vi "MainPr(Calculation)-37.vi"() -> ()   [LabVIEW 2013]
doc: "Main Program for Tracking\nThis VI Represents Front Panel and Control Buttons for Perform Tracking\nPlease, optimize the front panel for your own monitor resolution and needs"
uses:
  <vilib>/Utility/file.llb/Write To Spreadsheet File (DBL).vi
  <vilib>/vision/NI_Vision_Development_Module.lvlib
panel:
  out "error out":errorcluster
  in  "STOP Program":bool
  in  "Front Panel":T1(tab)
  in  "CurFrame":u32 max=9
  in  "Parameter 2":sgl format="%.2f"
  in  "Operator 2":T2(ring)
  out "2nd Movie (now disabled)":T3(plugin-control)
  out "1st Movie":T3(plugin-control)
  in  "Parameter":sgl format="%.2f"
  in  "Operator":T2(ring)
  in  "Index for thresholding 2":u8
  in  "Parameter 3":sgl format="%.2f"
  in  "Operator 3":T2(ring)
  in  "1/2 Channels":bool
  in  "Sigma #2":dbl min=0.1
  in  "Sigma":dbl min=0.1
  in  "Frame2":u32 max=499
  in  "Gray or Binarized?":bool
  out "2nd Movie Processed (now disabled)":T3(plugin-control)
  out "1st Movie Processed":T3(plugin-control)
  in  "Index for thresholding":u8 max=202
  in  "Keep Nega-\ntive Values?":bool
  out "Histogram of LoG \nprocessed image":T4(graph)
  out "Progress":u8(slide) scale=0.0..100.0
  in  "# Frame3":u32 max=499
  in  "Save pics (ex)":bool
  in  "Find ALL objects":bool
  out "Results on 1st Movie":T3(plugin-control)
  out "1st Filtering":T3(plugin-control)
  in  "Try my filters!":bool
  in  "# Erosion":i32=2
  in  "Connectivity":bool=TRUE
  in  "Min  Diam":dbl
  in  "Max  Diam":dbl min=12.0
  in  "Filter Tracks":bool
  out "Tracking progress":u8(slide) scale=0.0..100.0
  in  "Save data":bool
  in  "Save pictures":bool
  in  "Save movies":bool
  in  "Frame":u32 max=499
  in  "Delete Tracs":bool
  out "1st Filtered":T3(plugin-control)
  in  "dR max":dbl min=1.0
  out "1st Filtering (NN)":T3(plugin-control)
  in  "dR min":dbl min=0.0 max=10.0
  out "Raw #":i32
  out "Saved #":i32
  in  "Tracking Procedure":bool
  in  "Min TRK L":i32 min=2 max=498 step=1
  in  "Closing gaps":i32 min=1 max=498 step=1
  in  "% linearity":i32 min=1 max=100 step=1
  in  "Max angle":dbl min=0.0 max=89.0 step=1.0
  in  "Save problem trks":bool
  in  "Save pictures 2":bool
  in  "Delete Tracs 3":bool
  in  "Testing Frame":u32 min=68 max=76
  out "After":T3(plugin-control)
  out "Before":T3(plugin-control)
  in  "Tracks group":i32 min=0 max=515
  in  "Show Distributions":bool
  out "All Path Vel":T5(graph)
  out "All Instant Vel":T5(graph)
  out "mean Instant Vel":dbl format="%#_2g"
  out "StD Instant":dbl format="%#_2g"
  out "mean Path Vel":dbl format="%.2f"
  out "StD Path":dbl format="%.2f"
  in  "Bins":i32=10
  # "Two channels"
  # "*Two channels proce\nssing coming SOON"
  # "One channel"
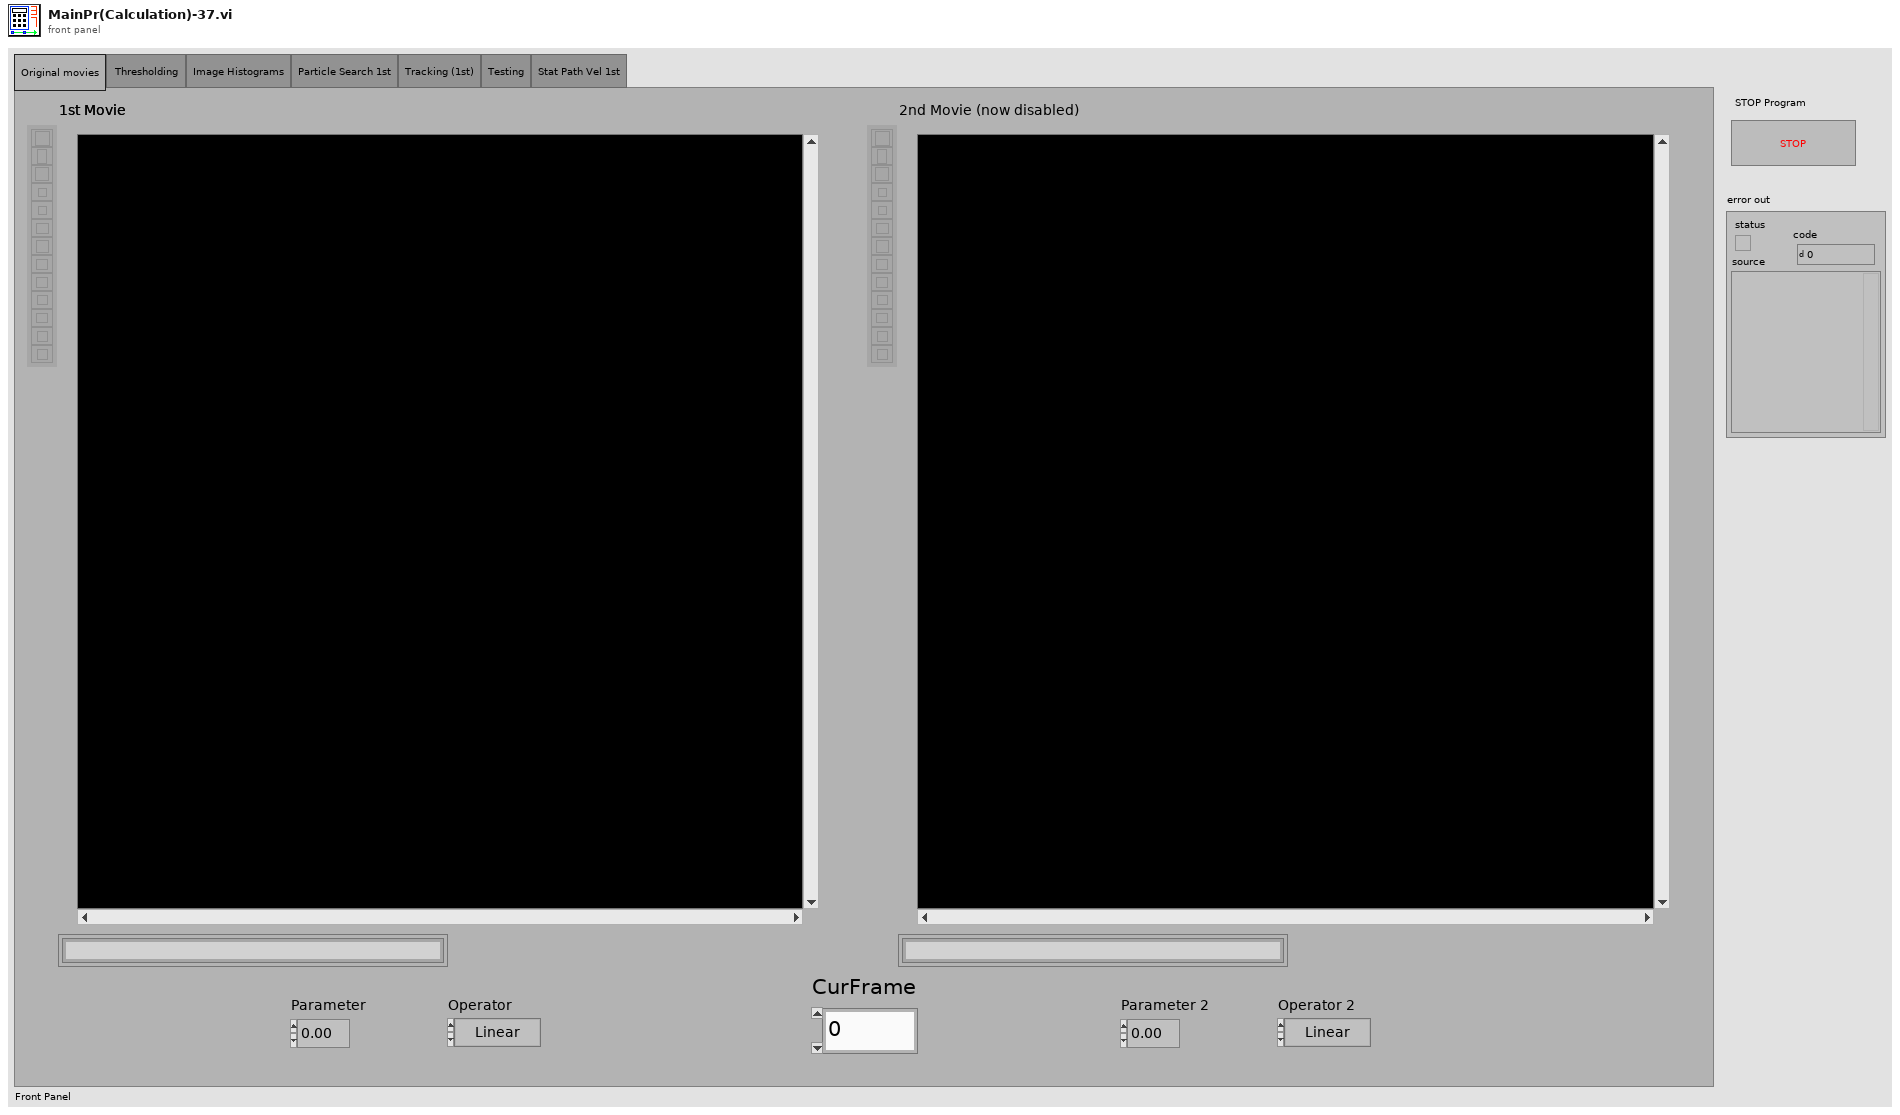
[diagram p1: front panel]
types:
  T1 = enum32{"Original movies", "Thresholding ", "Image Histograms", "Particle Search 1st", "Tracking (1st)", "Testing", "Stat Path Vel 1st"}
  T2 = enum32{"Linear", "Log", "Exp", "Square", "Square root", "Power X", "Power 1/X"}
  T3 = typedef "IMAQ Image.ctl" = refnum<image>
  T4 = cluster{"Starting Value":sgl, "Incremental Value":sgl, "Histogram":u32[]}
  T5 = cluster{"X Values":dbl[], "Histogram: h(x)":i32[]}
  T6 = enum8{"Enabled", "Disabled", "Disabled and Grayed Out"}
  T7 = cluster{"dR min ":dbl, "dR max ":dbl, "Closing gaps":i32, "Min TRK L":i32, "% linearity":i32, "Max angle":dbl, "Tracking progress":refnum<vi>}
  T8 = typedef "Image Type" = u32
  T9 = typedef "IMAQ AVI2 Refnum.ctl" = refnum<k20>
  T10 = cluster{"Intensity #1":sgl, "Operator #1":enum32{"Linear", "Log", "Exp", "Square", "Square root", "Power X", "Power 1/X"}, "Intensity #2":sgl, "Operator #2":enum32{"Linear", "Log", "Exp", "Square", "Square root", "Power X", "Power 1/X"}, "Sigma #1":dbl, "Sigma #2":dbl, "Index for \nthresholding":u8, "Index for \nthresholding 2":u8}
  T11 = typedef "Particle Parameters" = i32
  T12 = cluster{"X,Y":dbl[][], "Areas particles":dbl[][], "Particle Fil Setups":cluster{"Erosion":i32, "Connectivity ":bool, "Type of particle filter":cluster{"Measurement Parameter":T11, "Min  Diam":dbl, "Max  Diam":dbl, "Range":bool, "Range":bool}[]}, "Tracks, Coordinates":cluster{"(X,Y) Unmoved":dbl[][], "(X,Y,dX,dY) Dur 1 Frame":dbl[][], "(X,Y,dX,dY) W/t Problems":dbl[][], "(X,Y,dX,dY) NN filtered":dbl[][], "(X,Y,dX,dY) TH filtered":dbl[][], "Tracks":cluster{"Tracks":dbl[], "Start Pos":i32}[], "Tracks w/t Problems":cluster{"Tracks":dbl[], "Start Pos":i32}[]}}
  T13 = cluster{"Instant Vel 1st":dbl[], "Path Vel 1st ":dbl[], "Instant Vel 2nd  ":dbl[], "Path Vel 2nd":dbl[], "Time Measurments (Moving)":i32[], "Time Measurments (Unmoving) ":i16[]}
  T14 = cluster{"Before Grouped Tracks":cluster{"Tracks":dbl[][], "Start Pos":i32[], "Dot Statuses":i16[][]}[], "After Grouped Tracks":cluster{"Tracks":dbl[][], "Start Pos":i32[], "Dot Statuses":i16[][]}[], "Current\nGroup":i32}
  T15 = cluster{"Erosion":i32, "Connectivity ":bool, "Type of particle filter":cluster{"Measurement Parameter":T11, "Min  Diam":dbl, "Max  Diam":dbl, "Range":bool, "Range":bool}[]}
  T16 = cluster{"(X,Y) Unmoved":dbl[][], "(X,Y,dX,dY) Dur 1 Frame":dbl[][], "(X,Y,dX,dY) W/t Problems":dbl[][], "(X,Y,dX,dY) NN filtered":dbl[][], "(X,Y,dX,dY) TH filtered":dbl[][], "Tracks":cluster{"Tracks":dbl[], "Start Pos":i32}[], "Tracks w/t Problems":cluster{"Tracks":dbl[], "Start Pos":i32}[]}
  T17 = cluster{"Measurement Parameter":T11, "Min  Diam":dbl, "Max  Diam":dbl, "Range":bool, "Range":bool}[]
  T18 = cluster{"Points (X,Y)":dbl[], "Areas of points (X,Y)":dbl[]}[]
  T19 = cluster{"Points (X,Y)":dbl[], "Areas of points (X,Y)":dbl[]}
  T20 = cluster{"Area":dbl, "Number of Holes":dbl, "Bounding Rect":cluster{"Left":dbl, "Top":dbl, "Right":dbl, "Bottom":dbl}, "Center of Mass":cluster{"X":dbl, "Y":dbl}, "Orientation":dbl, "Dimensions":cluster{"Width":dbl, "Height":dbl}}[]
  T21 = cluster{"Tracks W/T Problems":dbl[], "Start Pos":i32}[]
  T22 = cluster{"Tracks":dbl[][], "Start Pos":i32[], "Dot Statuses":i16[][]}[]
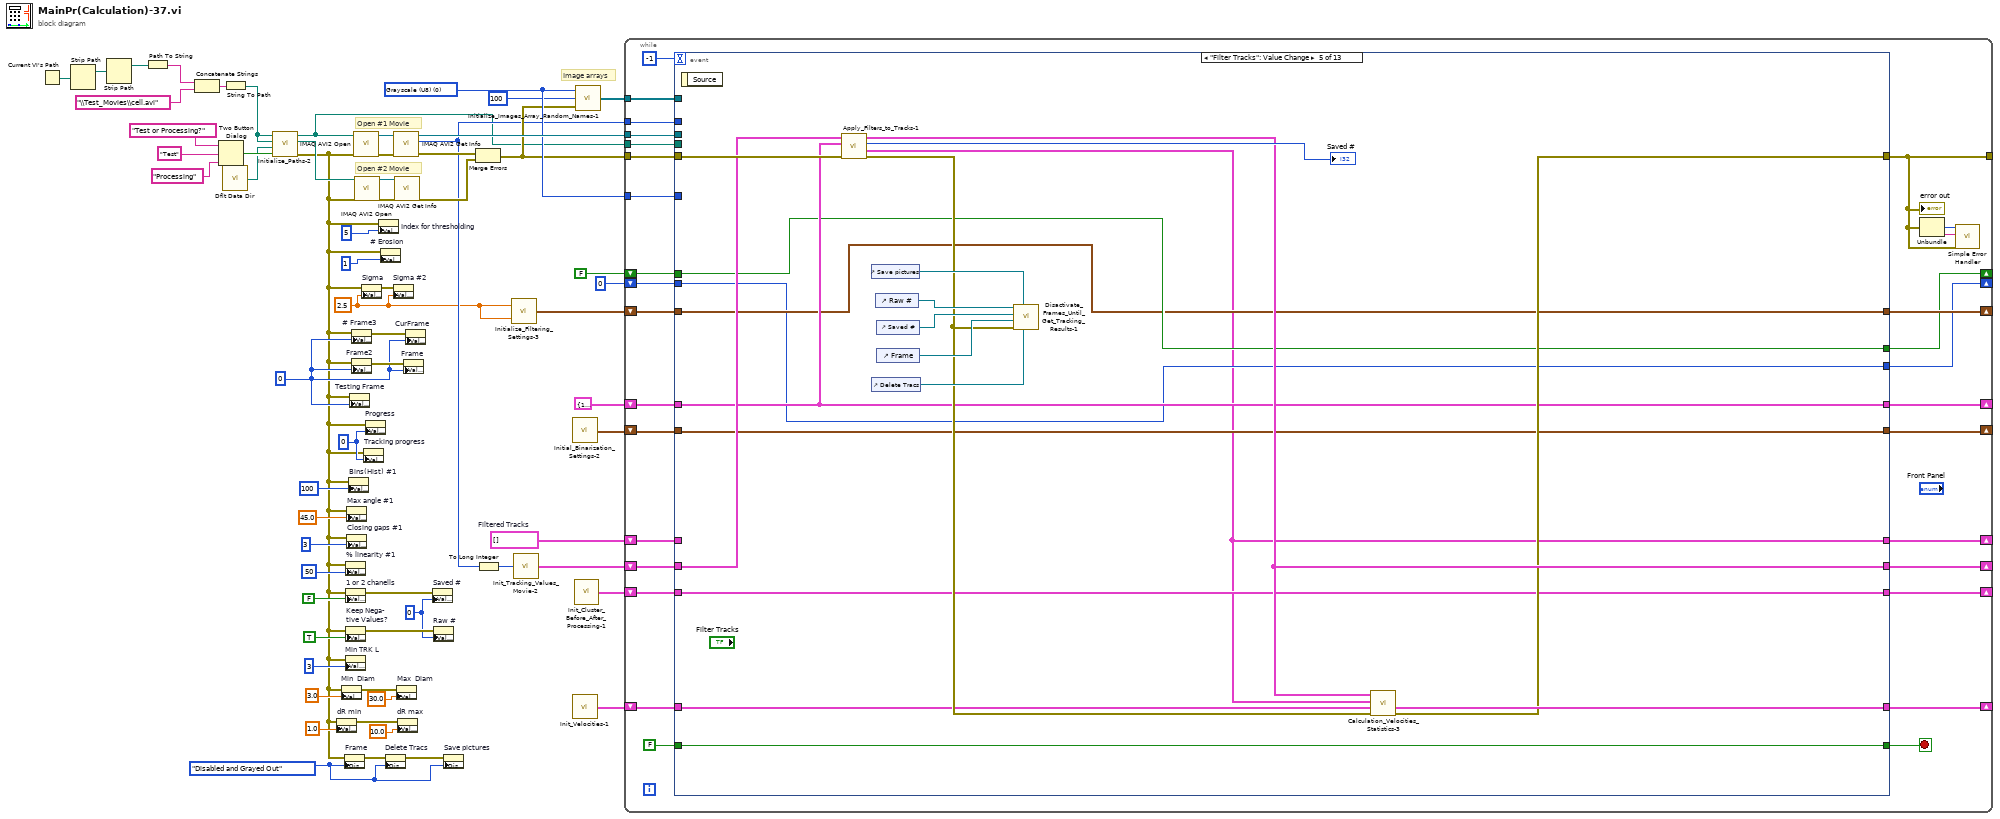
[diagram p0: block diagram]
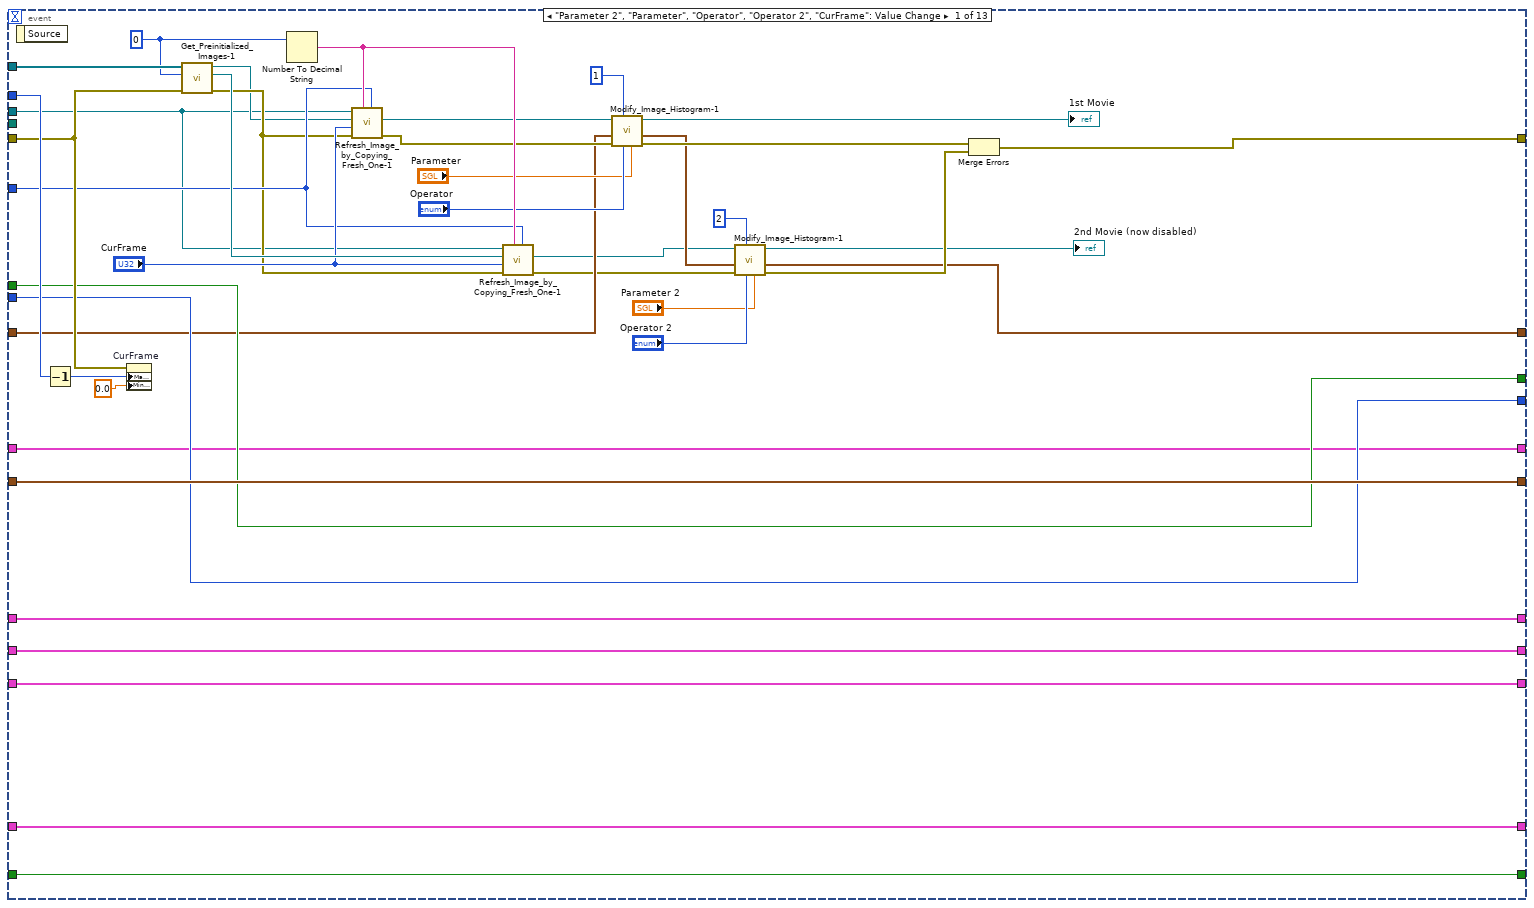
[diagram p2: hidden frame]
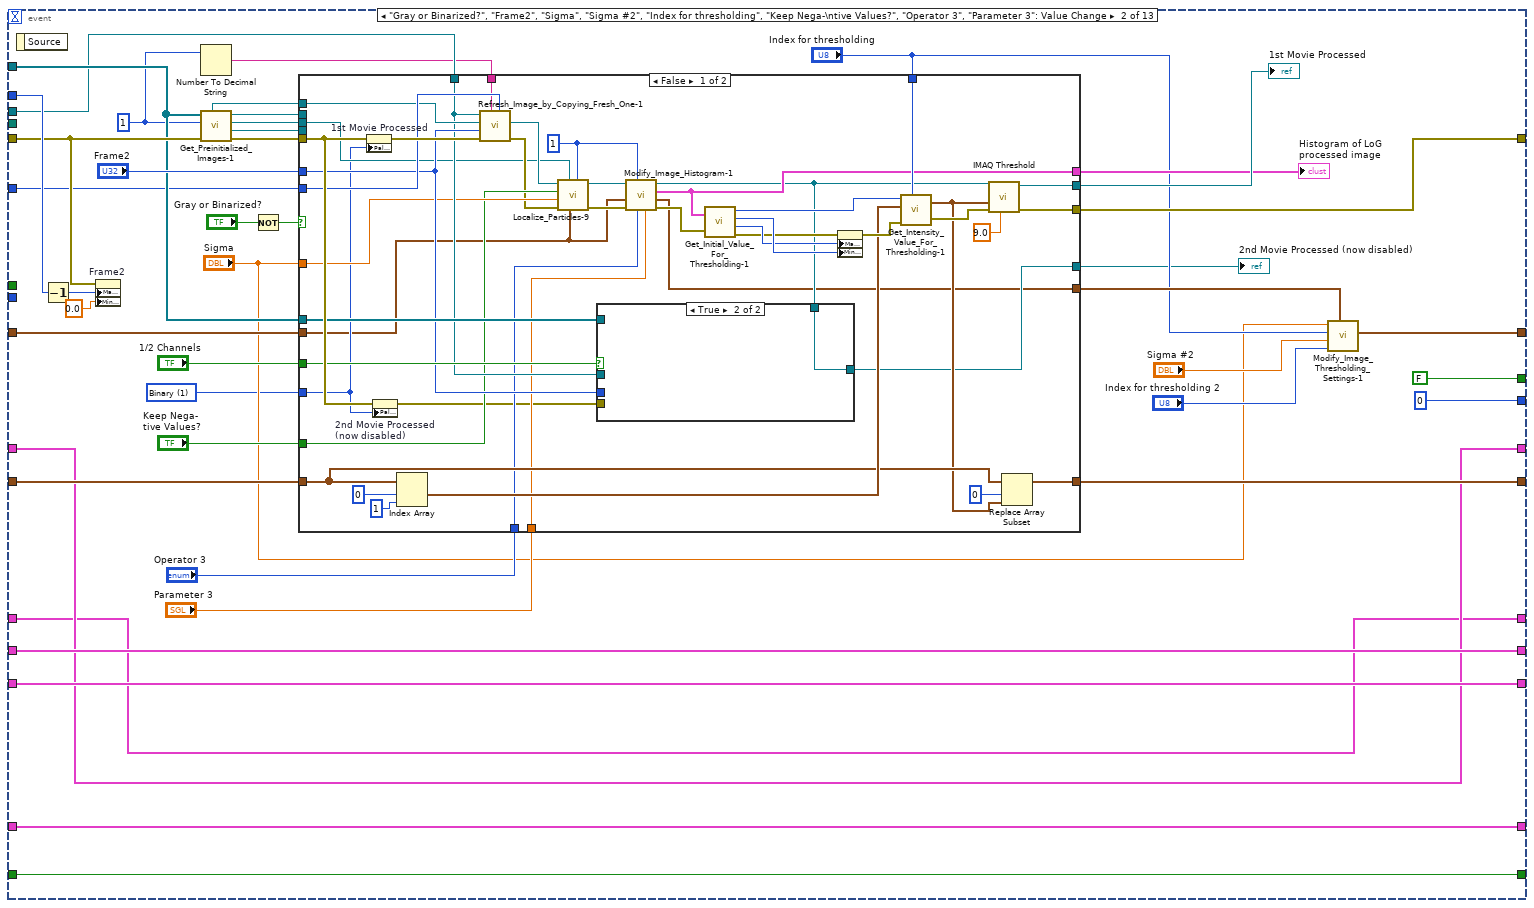
[diagram p3: hidden frame]
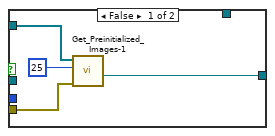
[diagram p4: hidden frame]
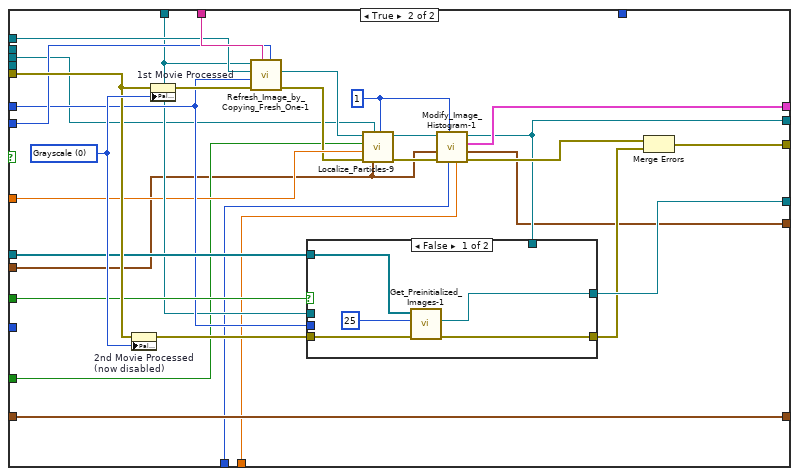
[diagram p5: hidden frame]
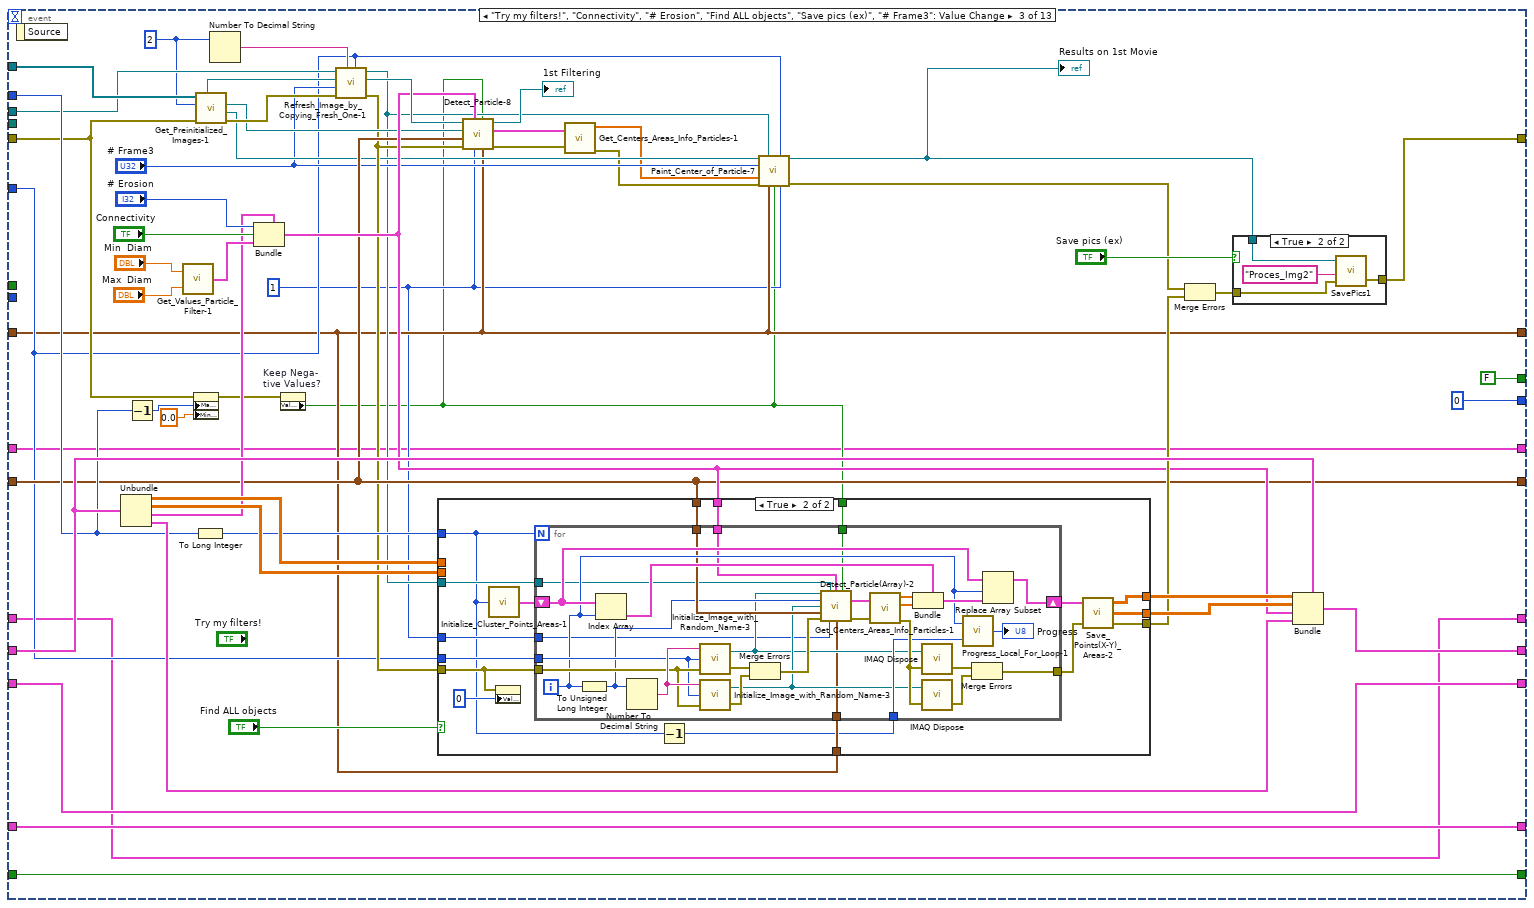
[diagram p7: hidden frame]
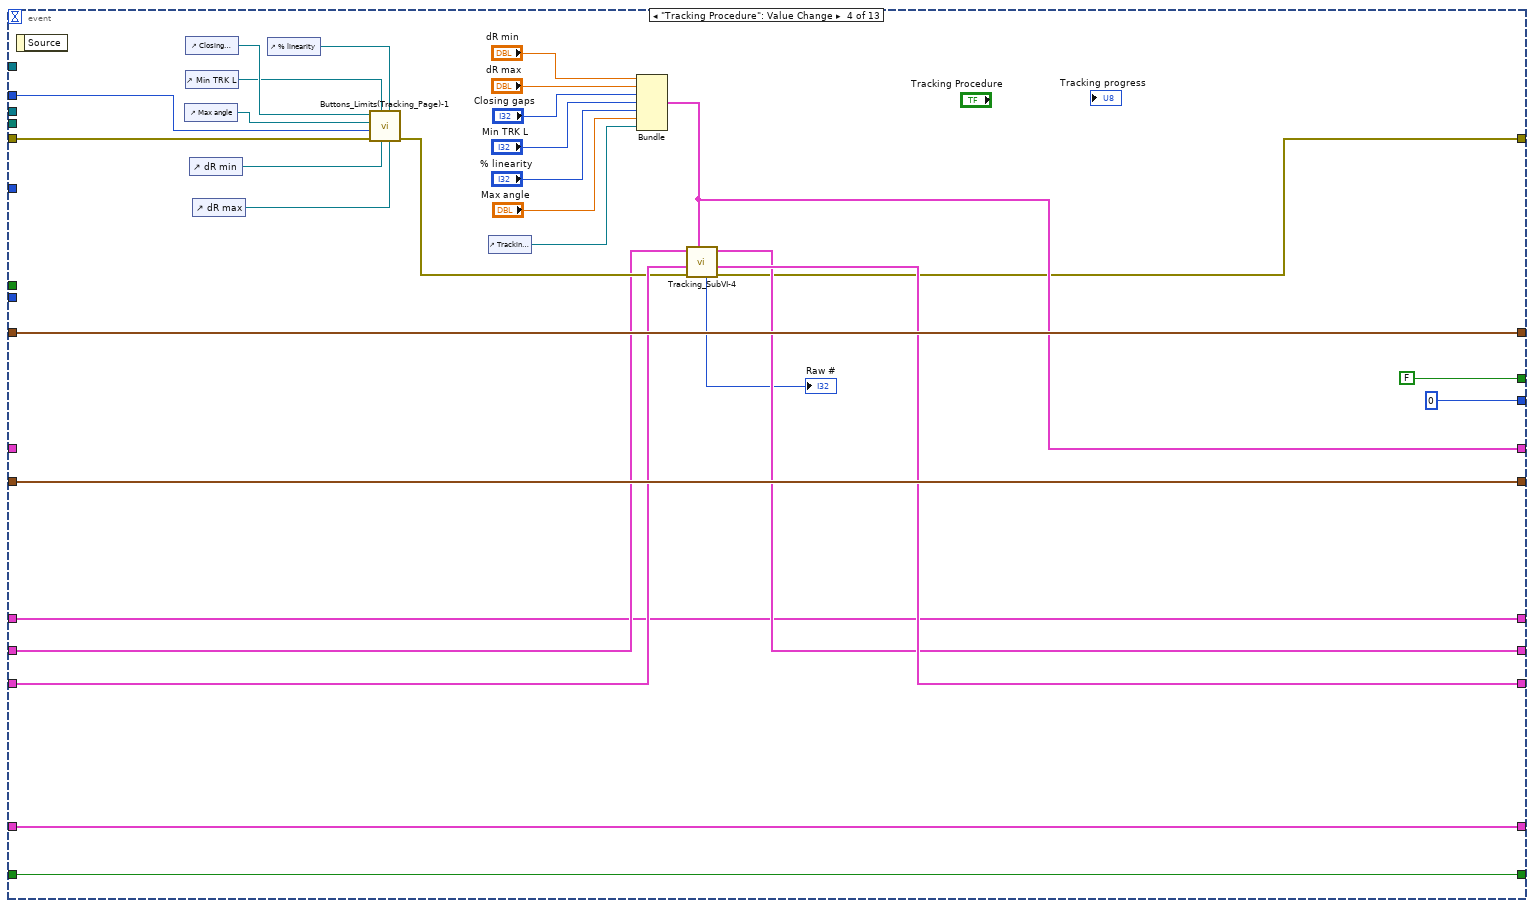
[diagram p10: hidden frame]
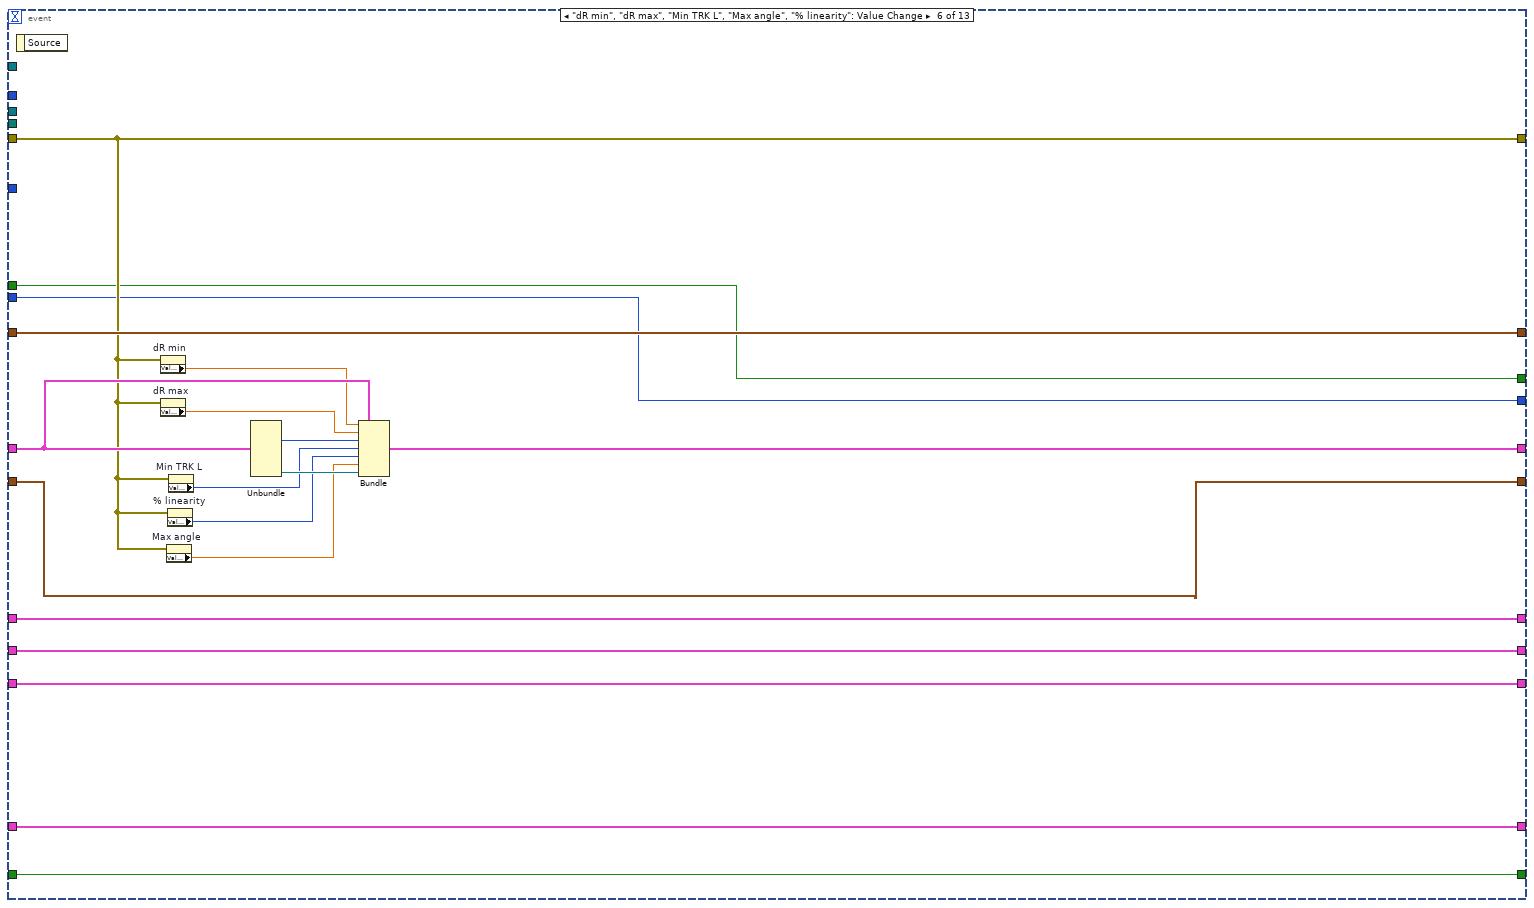
[diagram p11: hidden frame]
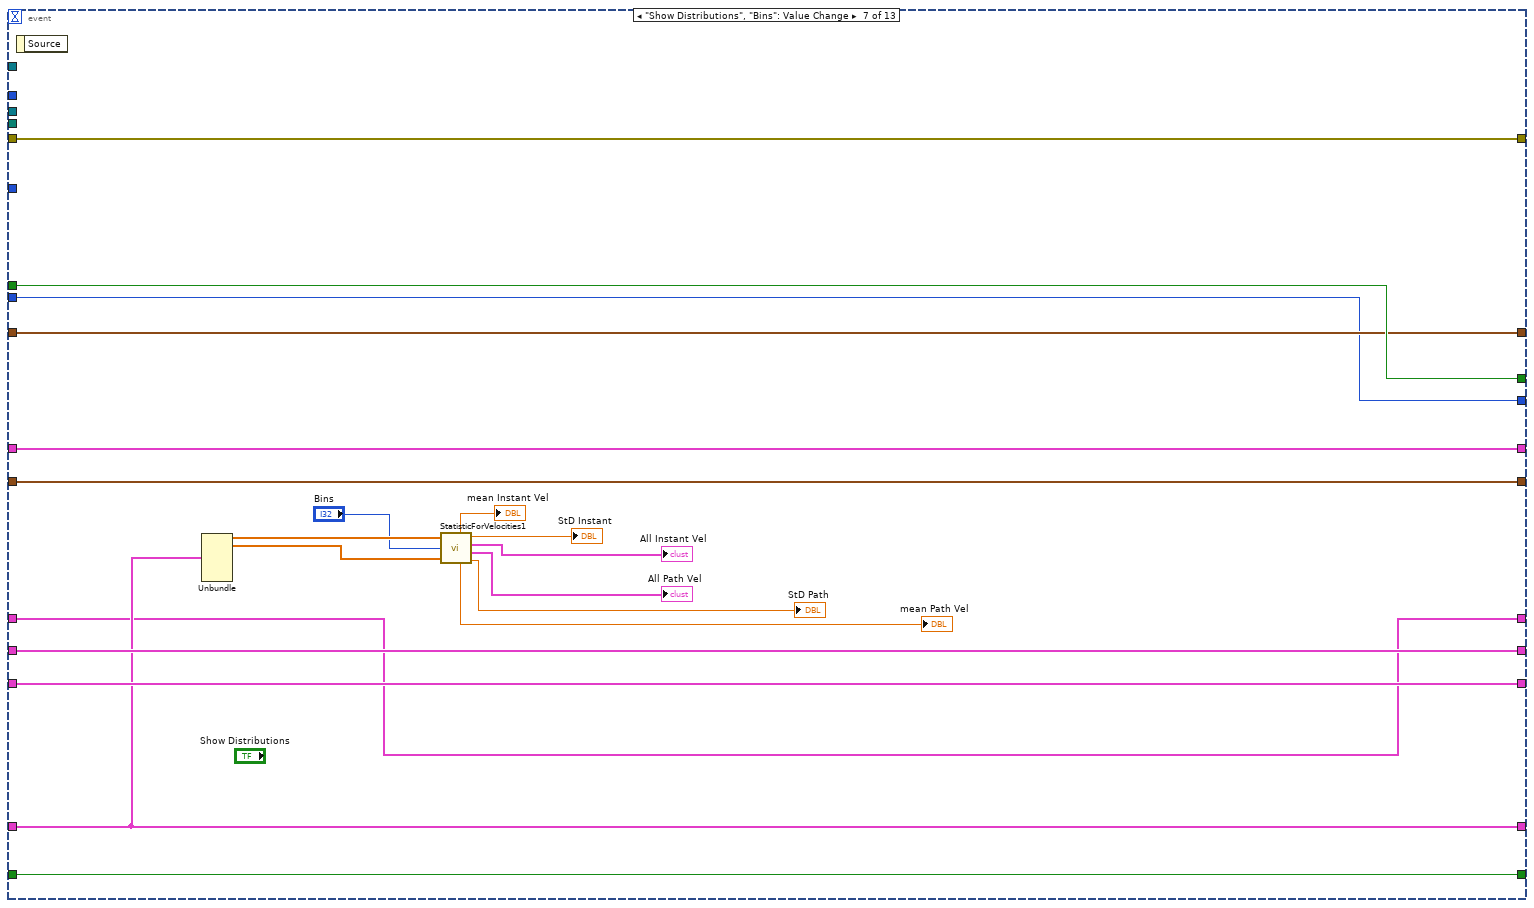
[diagram p12: hidden frame]
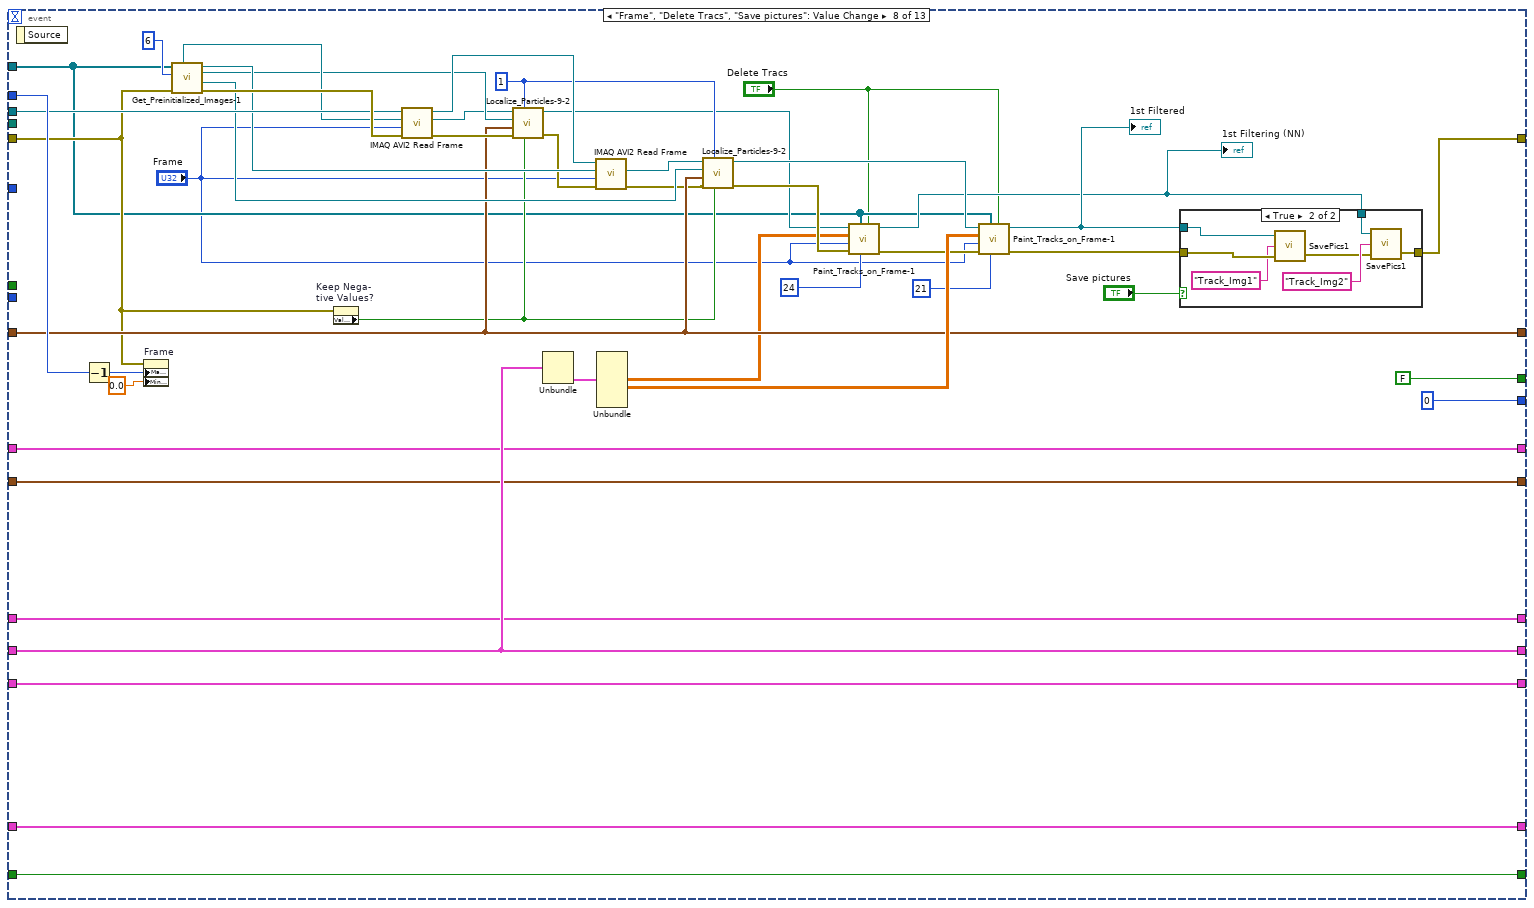
[diagram p13: hidden frame]
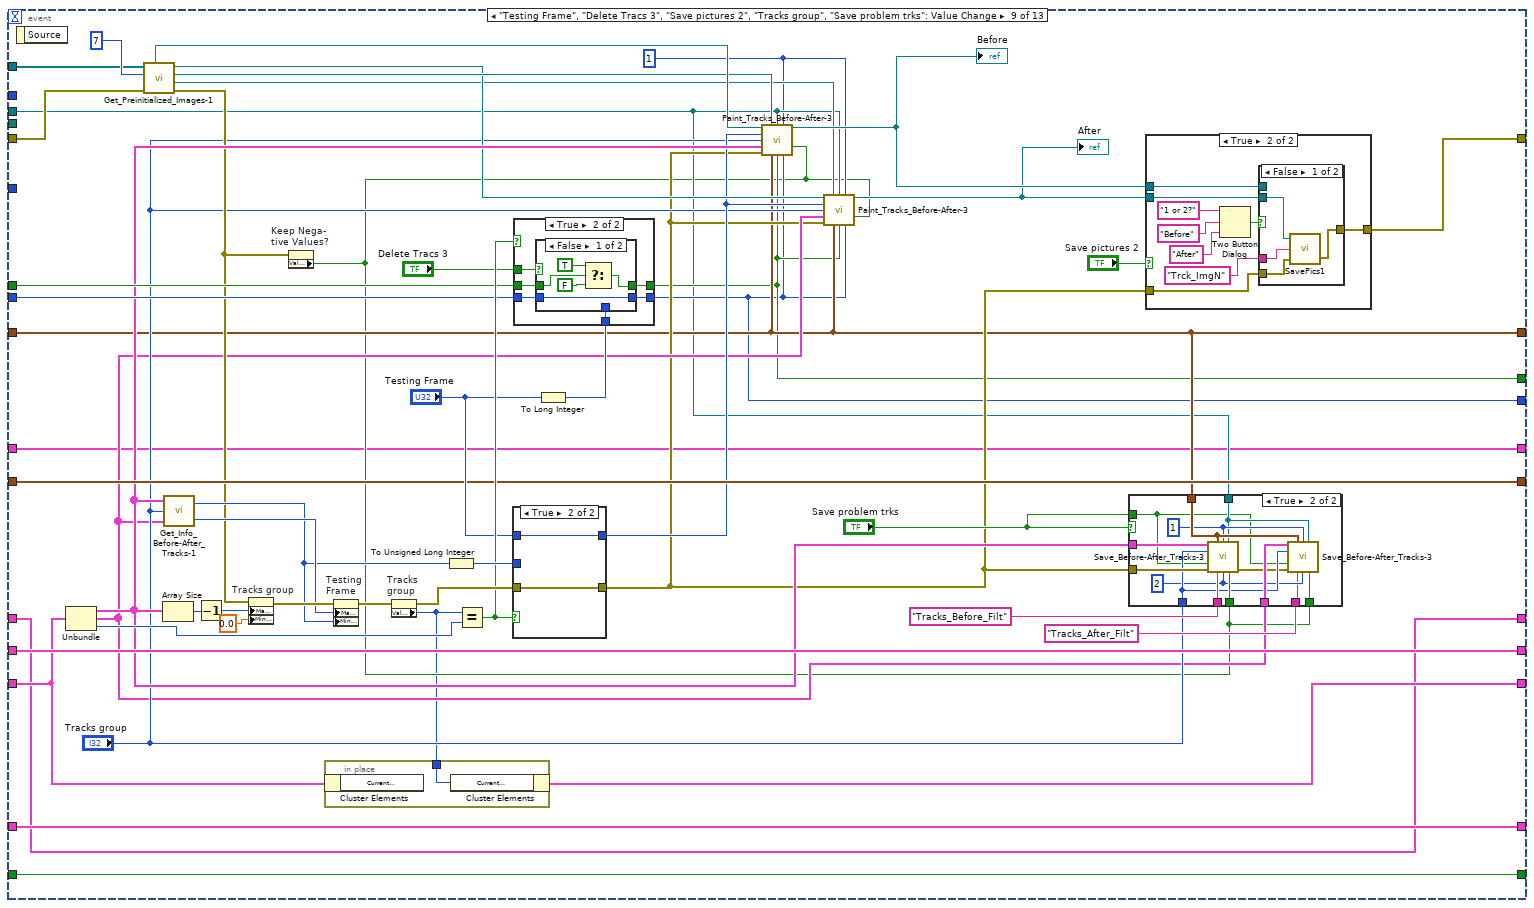
[diagram p15: hidden frame]
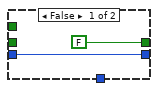
[diagram p16: hidden frame]
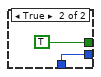
[diagram p17: hidden frame]
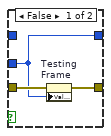
[diagram p19: hidden frame]
diagram:
  w1 = 0 ("Saved #")
  w4 = cluster{"Tracks":dbl[], "Start Pos":i32}[] []  # Filtered Tracks
  w5 = T6."Disabled and Grayed Out" ("Disabled")
  w14 = u32 0 ("Testing Frame")
  w27 = u8 0 ("Progress")
  w26 = 2.5 ("Sigma")
  w38 = T8 0 items=["Grayscale (U8)", "Grayscale (I16)", "Grayscale (SGL)", "Complex (CSG)", "RGB (U32)", "HSL (U32)", "RGB (U64)", "Grayscale (U16)"] ("Image Type")
  # "Image arrays"
  # "Open #2 Movie"
  # "Open #1 Movie"
  n1 = Current VI's Path() -> (path=w18:path)
  n2 = Strip Path(path=w18) -> (stripped path=w13:path)  [unwired: 1 out]
  n3 = Strip Path(path=w13) -> (stripped path=w12:path)  [unwired: 1 out]
  n4 = Path To String(path=w12) -> (string=w23:string)
  n5 = Concatenate Strings(w23, "\\Test_Movies\\cell.avi" ("string")) -> (w20:string)
  n6 = Two Button Dialog(message="Test or Processing?", 1:"Processing" ("F button name (\"Cancel\")"), 2:"Test" ("T button name (\"OK\")")) -> (T button?=w33:bool)
  n7 = call <vilib>:"Dflt Data Dir.vi"() -> ("App:Default Data Directory"=w21:path)
  n8 = String To Path(string=w20) -> (path=w19:path)
  n9 = call "Initialize_Paths-2.vi"("Test or Processing?"=w33, "start path"=w21, "AVI File Path #2"=w19, "AVI File Path #1"=w19) -> ("ERROR OUT"=w10:errorcluster, "AVI File Path #2 OUT"=w32:path, "AVI File Path #1 OUT"=w17:path)  [unwired: 1 out]
  n10 = property on="dR min" class="DigNum (strict)"(error in=w10, "Value"=1.0 ("dR min")) -> (error out=w42:errorcluster)  [unwired: 1 in, 1 out]
  n11 = property on="Min  Diam" class="DigNum (strict)"(error in=w10, "Value"=3.0 ("Min  Diam")) -> (error out=w45:errorcluster)  [unwired: 1 in, 1 out]
  n12 = property on="Frame" class="DigNum (strict)"(error in=w10, "DisabledEnum"=w5) -> (error out=w7:errorcluster)  [unwired: 1 in, 1 out]
  n13 = property on="Min TRK L" class="DigNum (strict)"(error in=w10, "Value"=3 ("Min TRK L")) -> ()  [unwired: 1 in, 2 out]
  n14 = property on="% linearity #1" class="DigNum (strict)"(error in=w10, "Value"=50 ("% linearity")) -> ()  [unwired: 1 in, 2 out]
  n15 = property on="1 or 2 chanells" class="Bool (strict)"(error in=w10, "Value"=FALSE) -> (error out=w3:errorcluster)  [unwired: 1 in, 1 out]
  n16 = property on="Keep Nega-\ntive Values?" class="Bool (strict)"(error in=w10, "Value"=TRUE ("Keep Nega-\ntive Values?")) -> (error out=w2:errorcluster)  [unwired: 1 in, 1 out]
  n17 = property on="Max angle #1" class="DigNum (strict)"(error in=w10, "Value"=45.0 ("Max angle")) -> ()  [unwired: 1 in, 2 out]
  n18 = property on="Closing gaps #1" class="DigNum (strict)"(error in=w10, "Value"=3 ("Closing gaps")) -> ()  [unwired: 1 in, 2 out]
  n19 = property on="Bins(Hist) #1" class="DigNum (strict)"(error in=w10, "Value"=100 ("Intervals")) -> ()  [unwired: 1 in, 2 out]
  n20 = property on="Testing Frame" class="DigNum (strict)"(error in=w10, "Value"=w14) -> ()  [unwired: 1 in, 2 out]
  n21 = property on="# Frame3" class="DigNum (strict)"(error in=w10, "Value"=w14) -> (error out=w16:errorcluster)  [unwired: 1 in, 1 out]
  n22 = property on="Frame2" class="DigNum (strict)"(error in=w10, "Value"=w14) -> (error out=w15:errorcluster)  [unwired: 1 in, 1 out]
  n23 = call "IMAQ AVI2 Open"("error in (no error)"=w10, "AVI File Path"=w17) -> ("error out"=w63:errorcluster, "AVI Refnum"=w64:T9)  [unwired: 8 in]
  n24 = call "IMAQ AVI2 Open"("error in (no error)"=w10, "AVI File Path"=w32) -> ("error out"=w62:errorcluster, "AVI Refnum"=w61:T9)  [unwired: 8 in]
  n25 = property on="Sigma" class="DigNum (strict)"(error in=w10, "Value"=w26) -> (error out=w56:errorcluster)  [unwired: 1 in, 1 out]
  n26 = property on="Tracking progress" class="Slide (strict)"(error in=w10, "Value"=w27) -> ()  [unwired: 1 in, 2 out]
  n27 = property on="Progress" class="Slide (strict)"(error in=w10, "Value"=w27) -> ()  [unwired: 1 in, 2 out]
  n28 = property on="Index for thresholding" class="DigNum (strict)"(error in=w10, "Value"=u8 5 ("Index for \nthresholding")) -> ()  [unwired: 1 in, 2 out]
  n29 = property on="# Erosion" class="DigNum (strict)"(error in=w10, "Value"=1 ("# Erosion")) -> ()  [unwired: 1 in, 2 out]
  n30 = property on="Delete Tracs" class="Bool"(error in=w7, "DisabledEnum"=w5) -> (error out=w6:errorcluster)  [unwired: 1 in, 1 out]
  n31 = property on="Sigma #2" class="DigNum (strict)"(error in=w56, "Value"=w26) -> ()  [unwired: 1 in, 2 out]
  n32 = call "IMAQ AVI2 Get Info"("error in (no error)"=w63, "AVI Refnum"=w64) -> ("error out"=w51:errorcluster, "Number of Frames"=w36:u32, "AVI Refnum (duplicate)"=w60:T9)  [unwired: 5 in, 2 out]
  n33 = call "IMAQ AVI2 Get Info"("error in (no error)"=w62, "AVI Refnum"=w61) -> ("error out"=w50:errorcluster)  [unwired: 5 in, 4 out]
  n34 = property on="Max  Diam" class="DigNum (strict)"(error in=w45, "Value"=30.0 ("Max  Diam")) -> ()  [unwired: 1 in, 2 out]
  n35 = property on="dR max" class="DigNum (strict)"(error in=w42, "Value"=10.0 ("dR max")) -> ()  [unwired: 1 in, 2 out]
  n36 = property on="Frame" class="DigNum (strict)"(error in=w15, "Value"=w14) -> ()  [unwired: 1 in, 2 out]
  n37 = property on="CurFrame" class="DigNum (strict)"(error in=w16, "Value"=w14) -> ()  [unwired: 1 in, 2 out]
  n38 = property on="Saved #" class="DigNum (strict)"(error in=w3, "Value"=w1) -> ()  [unwired: 1 in, 2 out]
  n39 = property on="Raw #" class="DigNum (strict)"(error in=w2, "Value"=w1) -> ()  [unwired: 1 in, 2 out]
  n40 = property on="Save pictures" class="Bool"(error in=w6, "DisabledEnum"=w5) -> ()  [unwired: 1 in, 2 out]
  n41 = Merge Errors(w51, w50) -> (w37:errorcluster)
  n42 = To Long Integer(number=w36) -> (32bit integer=w9:i32)
  n43 = call "Initialize_Filtering_Settings-3.vi"("Sigma #2"=w26, "Sigma #1"=w26) -> ("[OUT] Filtering Settings"=w25:T10)
  n44 = call "Init_Tracking_Values_Movie-2.vi"("[IN] # Frames"=w9) -> ("[OUT] Movie Values\n(Empty Cluster)"=w8:T12)
  n45 = call "Initial_Binarization_Settings-2.vi"() -> ("Binarization Settings"=w40:cluster{"MinBin2":sgl, "MaxBin2":sgl}[])
  n46 = call "Init_Velocities-1.vi"() -> ("[OUT] Cluster with Velocities"=w48:T13)
  n47 = call "Init_Cluster_Before_After_Processing-1.vi"() -> ("[OUT] Before-After"=w31:T14)
  n48 = call "Initialize_Images_Array_Random_Names-1.vi"("error IN"=w37, "# Pics"=100, "Image Type"=w38) -> ("Images Array"=w35:T3[])
  n49 = while {
    tunnel: w37 -> [w88]
    tunnel: w36 -> [w91]
    tunnel: [w83] -> _
    tunnel: w60 -> [w92]
    shift-right: [w86] -> _
    shift-left: w8 -> [w87]
    shift-right: [w84] -> _
    shift-left: w48 -> [w85]
    shift-right: [w81] -> _
    shift-left: w31 -> [w82]
    shift-right: [w79] -> _
    shift-left: w40 -> [w80]
    shift-right: [w77] -> _
    shift-left: w25 -> [w78]
    tunnel: w38 -> [w76]
    tunnel: w35 -> [w75]
    shift-right: [w73] -> _
    shift-left: FALSE ("Delete Tracs 3") -> [w74]
    shift-right: [w71] -> _
    shift-left: 0 -> [w72]
    tunnel: w17 -> [w69]
    shift-right: [w68] -> _
    shift-left: T7 {"dR min "=1.0, "dR max "=10.0, "Closing gaps"=3, "Min TRK L"=3, "% linearity"=50, "Max angle"=46.0, "Tracking progress"=refnum} -> [w67]
    shift-right: [w65] -> _
    shift-left: w4 -> [w66]
    stop <- w94 stop-if-true
    n50 = event shown="[4] \"Filter Tracks\": Value Change" {
      selector: _ -> [_ _ _ _ _ _ _ _ _ _ _ _ _]
      dyn-events: _ -> [_ _ _ _ _ _ _ _ _ _ _ _ _]
      timeout: -1 -> [_ _ _ _ _ _ _ _ _ _ _ _ _]
      tunnel: [w97 w138 w266 w385 w413 w437 w451 w477 w524 w625 w645 "STOP Program" w697] -> w94
      tunnel: w92 -> [w115 w159 w291 _ _ _ _ w499 w528 w633 _ w684 _]
      tunnel: w88 -> [w126 w161 w295 w401 w425 w431 w464 w475 w562 w636 w653 w683 w705]
      tunnel: w91 -> [w127 w163 w297 w400 _ _ _ w502 _ _ _ _ _]
      tunnel: [w130 w167 w309 w378 w412 w431 w464 w509 w560 w626 w646 w679 w705] -> w83
      tunnel: w87 -> [w134 w169 w317 w380 w424 w440 w459 w508 w567 w640 w656 w693 w704]
      tunnel: [w134 w169 w314 w379 w415 w440 w459 w508 w567 w640 w656 w693 w704] -> w86
      tunnel: w85 -> [w131 w172 w311 w375 w416 w438 w457 w505 w569 w641 w655 w691 w703]
      tunnel: [w131 w172 w311 w375 w414 w438 w457 w505 w569 w641 w655 w691 w703] -> w84
      tunnel: w82 -> [w129 w168 w304 w383 w411 w439 w458 w503 w523 w638 w652 w690 w702]
      tunnel: [w129 w168 w304 w381 w411 w439 w458 w503 w521 w638 w652 w690 w702] -> w81
      tunnel: w80 -> [w128 w166 w282 w404 w410 w429 w460 w501 w543 w630 w651 w689 w701]
      tunnel: [w128 w165 w282 w404 w410 w429 w460 w501 w543 w630 w651 w689 w701] -> w79
      tunnel: w78 -> [w108 w164 w270 w388 w407 w443 w462 w482 w531 w629 w650 w688 w700]
      tunnel: [w98 w141 w270 w388 w407 w443 w462 w482 w531 w629 w650 w688 w700] -> w77
      tunnel: w76 -> [w120 w156 w271 _ _ _ _ _ _ _ _ _ _]
      tunnel: w75 -> [w125 w160 w294 _ _ _ _ w467 w556 _ _ w687 _]
      tunnel: w74 -> [w117 _ _ _ w408 w427 w463 _ w549 w628 w648 w686 w699]
      tunnel: [w117 FALSE ("Delete Tracs 3") FALSE ("Delete Tracs 3") FALSE ("Delete Tracs 3") w408 w427 w463 FALSE ("Delete Tracs 3") w530 w628 w648 w686 w699] -> w73
      tunnel: w72 -> [w116 _ _ _ w406 w426 w461 _ w548 w627 w647 w685 w698]
      tunnel: [w116 0 0 0 w406 w426 w461 0 w529 w627 w647 w685 w698] -> w71
      tunnel: FALSE ("STOP Program") -> [w97 w138 w266 w385 w413 w437 w451 w477 w524 w625 w645 _ w697]
      tunnel: w69 -> [_ _ _ _ _ _ _ _ _ _ w644 _ _]
      tunnel: [w96 w136 w265 w384 w409 w428 w446 w476 w520 w624 w643 w678 w696] -> w68
      tunnel: w67 -> [w96 w136 w265 _ w409 w444 w446 w476 w520 w624 w643 w678 w696]
      tunnel: w66 -> [w95 w135 w264 w376 _ w441 w445 w474 w519 w623 w642 w677 w695]
      tunnel: [w95 w135 w264 w376 w405 w441 w445 w474 w519 w623 w642 w677 w695] -> w65
      event "Parameter 2", "Parameter", "Operator", "Operator 2", "CurFrame": Value Change {
        w124 = i8 0 ("[IN] Number of event")
        n51 = event-data() -> ()  [unwired: 1 in, 1 out]
        n52 = Decrement(x=w127) -> (x-1=w132:u32)
        n53 = property on="CurFrame" class="DigNum (strict)"(error in=w126, "Maximum"=w132, "Minimum"=0.0 ("Data Entry Limits:Minimum")) -> ()  [unwired: 1 in, 2 out]
        n54 = call "Get_Preinitialized_Images-1.vi"("error IN"=w126, "[IN] Number of event"=w124, "[IN] Images Array"=w125) -> ("error OUT"=w119:errorcluster, "[OUT] Processed Image #1"=w123:T3, "[OUT] Source Image #2"=w118:T3)  [unwired: 1 in, 2 out]
        n55 = Number To Decimal String(number=w124) -> (decimal integer string=w121:string)  [unwired: 1 in]
        n56 = call "Refresh_Image_by_Copying_Fresh_One-1.vi"("[IN] Image Type"=w120, "[IN] Unique ID\n(# of Event)"=w121, "error IN"=w119, "Frame Number"="CurFrame", "[IN] Preinitialized Image"=w118, "[IN] AVI Refnum"=w115) -> ("error OUT"=w113:errorcluster, "[OUT] Frame"=w114:T3)  [unwired: 1 in, 1 out]
        n57 = call "Refresh_Image_by_Copying_Fresh_One-1.vi"("[IN] Image Type"=w120, "[IN] Unique ID\n(# of Event)"=w121, "error IN"=w119, "Frame Number"="CurFrame", "[IN] Preinitialized Image"=w123, "[IN] AVI Refnum"=w115) -> ("error OUT"=w106:errorcluster, "[OUT] Frame"=w104:T3)  [unwired: 1 in, 1 out]
        n58 = call "Modify_Image_Histogram-1.vi"("[IN] Parameter"="Parameter", "[IN] Operator"="Operator", "# channel"=u8 1, "error IN"=w113, "[IN] Filtering Settings"=w108, "[IN] LoG Processed Image"=w114) -> ("error OUT"=w111:errorcluster, "[OUT] Filtering Settings"=w105:T10, "[OUT] Histogram Modified Image"=→"1st Movie":T3)  [unwired: 2 in, 1 out]
        n59 = call "Modify_Image_Histogram-1.vi"("[IN] Parameter"="Parameter 2", "[IN] Operator"="Operator 2", "# channel"=u8 2, "error IN"=w106, "[IN] Filtering Settings"=w105, "[IN] LoG Processed Image"=w104) -> ("error OUT"=w100:errorcluster, "[OUT] Filtering Settings"=w98:T10, "[OUT] Histogram Modified Image"=→"2nd Movie (now disabled)":T3)  [unwired: 2 in, 1 out]
        n60 = Merge Errors(w111, w100) -> (w130:errorcluster)
      }
      event "Gray or Binarized?", "Frame2", "Sigma", "Sigma #2", "Index for thresholding", "Keep Nega-\ntive Values?", "Operator 3", "Parameter 3": Value Change {
        w139 = u32 1 items=["Grayscale", "Binary", "Gradient", "Rainbow", "Temperature", "User Defined"] ("Palette:Palette Type")
        w157 = i8 1 ("[IN] Number of event")
        n61 = event-data() -> ()  [unwired: 1 in, 1 out]
        n62 = Decrement(x=w163) -> (x-1=w173:u32)
        n63 = property on="Frame2" class="DigNum (strict)"(error in=w161, "Maximum"=w173, "Minimum"=0.0 ("Data Entry Limits:Minimum")) -> ()  [unwired: 1 in, 2 out]
        n64 = Number To Decimal String(number=w157) -> (decimal integer string=w155:string)  [unwired: 1 in]
        n65 = call "Get_Preinitialized_Images-1.vi"("error IN"=w161, "[IN] Number of event"=w157, "[IN] Images Array"=w160) -> ("error OUT"=w158:errorcluster, "[OUT] Processed Image #2"=w151:T3, "[OUT] Processed Image #1"=w152:T3, "[OUT] Source Image #2"=w153:T3, "[OUT] Source Image #1"=w154:T3)  [unwired: 1 in]
        n66 = Not(x="Gray or Binarized?") -> (.not. x?=w176:bool)
        n67 = case shown="False" w176 {
          tunnel: w158 -> [w221 w255]
          tunnel: [w204 w254] -> w167
          tunnel: [w202 w251] -> w137
          tunnel: [w220 w230] -> w175
          tunnel: "Sigma" -> [w193 w240]
          tunnel: [w185 w232] -> w171
          tunnel: "Frame2" -> [w197 w243]
          tunnel: "1/2 Channels" -> [w219 w252]
          tunnel: "Index for thresholding" -> [w205 _]
          tunnel: w166 -> [w208 w249]
          tunnel: [w207 w249] -> w165
          tunnel: w164 -> [w186 w234]
          tunnel: w160 -> [w203 w248]
          tunnel: w159 -> [w196 w242]
          tunnel: w156 -> [w200 w245]
          tunnel: w155 -> [w199 w247]
          tunnel: w154 -> [w198 w244]
          tunnel: w153 -> [_ _]
          tunnel: w152 -> [w190 w238]
          tunnel: w151 -> [_ _]
          tunnel: "Keep Nega-\ntive Values?" -> [w192 w237]
          tunnel: [w182 w229] -> w145
          tunnel: "Parameter 3" -> [w179 w228]
          tunnel: "Operator 3" -> [w180 w227]
          tunnel: w139 -> [w189 _]
          frame False {
            w181 = u8 1 ("# channel")
            n68 = property on="1st Movie Processed" class="ImageControl"(error in=w221, "Palette Type"=w189) -> (error out=w201:errorcluster)  [unwired: 1 in, 1 out]
            n69 = property on="2nd Movie Processed (now disabled)" class="ImageControl"(error in=w221, "Palette Type"=w189) -> (error out=w178:errorcluster)  [unwired: 1 in, 1 out]
            n70 = Index Array(array=w208, index #1=0 ("index"), index #2=1 ("index")) -> (element #1=w209:cluster{"MinBin2":sgl, "MaxBin2":sgl})  [unwired: 1 out]
            n71 = call "Refresh_Image_by_Copying_Fresh_One-1.vi"("[IN] Image Type"=w200, "[IN] Unique ID\n(# of Event)"=w199, "error IN"=w201, "Frame Number"=w197, "[IN] Preinitialized Image"=w198, "[IN] AVI Refnum"=w196) -> ("error OUT"=w191:errorcluster, "[OUT] Frame"=w194:T3)  [unwired: 1 in, 1 out]
            n72 = call "Localize_Particles-9.vi"("# channel"=w181, "[IN] Filtering Settings"=w186, "[IN] Destination Image"=w190, "error IN"=w191, "[IN] Sigma"=w193, "Keep Nega-\ntive Values?"=w192, "[IN] Frame"=w194) -> ("error OUT"=w187:errorcluster, "[OUT] LoG Processed Image"=w188:T3)  [unwired: 1 in, 1 out]
            n73 = call "Modify_Image_Histogram-1.vi"("[IN] Parameter"=w179, "[IN] Operator"=w180, "# channel"=w181, "error IN"=w187, "[IN] Filtering Settings"=w186, "[IN] LoG Processed Image"=w188) -> ("error OUT"=w183:errorcluster, "[OUT] Filtering Settings"=w182:T10, "[OUT] Histogram"=w185:T4, "[OUT] Histogram Modified Image"=w184:T3)  [unwired: 2 in]
            n74 = case shown="True" w219 {
              tunnel: w178 -> [w225 _]
              tunnel: w196 -> [_ _]
              tunnel: w197 -> [_ _]
              tunnel: [w224 w226] -> w202
              tunnel: w203 -> [w223 _]
              tunnel: w184 -> [_ w226]
              frame False {
                n75 = call "Get_Preinitialized_Images-1.vi"("error IN"=w225, "[IN] Number of event"=i8 25, "[IN] Images Array"=w223) -> ("[OUT] Processed Image #2"=w224:T3)  [unwired: 1 in, 4 out]
              }
              frame True {
              }
            }
            n76 = call "Get_Initial_Value_For_Thresholding-1.vi"("[IN] Histogram Graph"=w185, "error IN"=w183) -> ("[OUT] Index of starting \npoint for thresholding"=w218:i32, "[OUT] Minimal index for \nthresholding (negative)"=w217:i32, "[OUT] Maximal index \nfor thresholding"=w216:i32, "error OUT"=w195:errorcluster)
            n77 = property on="Index for thresholding" class="DigNum (strict)"(error in=w195, "Maximum"=w216, "Minimum"=w217) -> (error out=w215:errorcluster)  [unwired: 1 in, 1 out]
            n78 = call "Get_Intensity_Value_For_Thresholding-1.vi"("[IN] Index of starting \npoint for thresholding"=w218, "[IN] Thresholding range"=w209, "error IN"=w215, "[IN] Index for \nthresholding"=w205) -> ("[OUT] Thresholding range"=w206:cluster{"Lower value":sgl, "Upper value":sgl}, "error OUT"=w212:errorcluster)  [unwired: 1 in]
            n79 = call "IMAQ Threshold"("Replace Value"=sgl 9.0, "error in (no error)"=w212, "Range"=w206, "Image Src"=w184) -> ("error out"=w204:errorcluster, "Image Dst Out"=w220:T3)  [unwired: 6 in]
            n80 = Replace Array Subset(array=w208, new element=w206, index=0) -> (w207:cluster{"MinBin2":sgl, "MaxBin2":sgl}[])
          }
          frame True {
            w233 = u8 1 ("# channel")
            w256 = u32 0 items=["Grayscale", "Binary", "Gradient", "Rainbow", "Temperature", "User Defined"] ("Palette:Palette Type")
            n81 = property on="2nd Movie Processed (now disabled)" class="ImageControl"(error in=w255, "Palette Type"=w256) -> (error out=w253:errorcluster)  [unwired: 1 in, 1 out]
            n82 = property on="1st Movie Processed" class="ImageControl"(error in=w255, "Palette Type"=w256) -> (error out=w246:errorcluster)  [unwired: 1 in, 1 out]
            n83 = call "Refresh_Image_by_Copying_Fresh_One-1.vi"("[IN] Image Type"=w245, "[IN] Unique ID\n(# of Event)"=w247, "error IN"=w246, "Frame Number"=w243, "[IN] Preinitialized Image"=w244, "[IN] AVI Refnum"=w242) -> ("error OUT"=w239:errorcluster, "[OUT] Frame"=w241:T3)  [unwired: 1 in, 1 out]
            n84 = call "Localize_Particles-9.vi"("# channel"=w233, "[IN] Filtering Settings"=w234, "[IN] Destination Image"=w238, "error IN"=w239, "[IN] Sigma"=w240, "Keep Nega-\ntive Values?"=w237, "[IN] Frame"=w241) -> ("error OUT"=w236:errorcluster, "[OUT] LoG Processed Image"=w235:T3)  [unwired: 1 in, 1 out]
            n85 = call "Modify_Image_Histogram-1.vi"("[IN] Parameter"=w228, "[IN] Operator"=w227, "# channel"=w233, "error IN"=w236, "[IN] Filtering Settings"=w234, "[IN] LoG Processed Image"=w235) -> ("error OUT"=w231:errorcluster, "[OUT] Filtering Settings"=w229:T10, "[OUT] Histogram"=w232:T4, "[OUT] Histogram Modified Image"=w230:T3)  [unwired: 2 in]
            n86 = case shown="False" w252 {
              tunnel: w253 -> [w261 w263]
              tunnel: w230 -> [_ w262]
              tunnel: w242 -> [_ _]
              tunnel: w243 -> [_ _]
              tunnel: [w259 w262] -> w251
              tunnel: [w260 w263] -> w250
              tunnel: w248 -> [w257 _]
              frame False {
                n87 = call "Get_Preinitialized_Images-1.vi"("error IN"=w261, "[IN] Number of event"=i8 25, "[IN] Images Array"=w257) -> ("error OUT"=w260:errorcluster, "[OUT] Processed Image #1"=w259:T3)  [unwired: 1 in, 3 out]
              }
              frame True {
              }
            }
            n88 = Merge Errors(w231, w250) -> (w254:errorcluster)
          }
        }
        "1st Movie Processed" <- w175
        "2nd Movie Processed (now disabled)" <- w137
        "Histogram of LoG \nprocessed image" <- w171
        n89 = call "Modify_Image_Thresholding_Settings-1.vi"("[IN] Filtering Settings"=w145, "[IN] Index for thresholding 2"="Index for thresholding 2", "[IN] Sigma #2"="Sigma #2", "[IN] Index for thresholding"="Index for thresholding", "[IN] Sigma"="Sigma") -> ("[OUT] Filtering Settings"=w141:T10)  [unwired: 3 in]
      }
      event "Try my filters!", "Connectivity", "# Erosion", "Find ALL objects", "Save pics (ex)", "# Frame3": Value Change {
        w290 = i8 2 ("[IN] Number of event")
        w269 = u8 1 ("# Channel")
        n90 = event-data() -> ()  [unwired: 1 in, 1 out]
        n91 = Unbundle(w317) -> ("X,Y"=w318:dbl[][], "Areas particles"=w305:dbl[][], "Particle Fil Setups"=w300:T15, "Tracks, Coordinates"=w316:T16)
        n92 = Decrement(x=w297) -> (x-1=w312:u32)
        n93 = call "Get_Values_Particle_Filter-1.vi"("Max  Diam"="Max  Diam", "Min  Diam"="Min  Diam") -> ("type of filters\nparticles search"=w301:T17)
        n94 = property on="# Frame3" class="DigNum (strict)"(error in=w295, "Maximum"=w312, "Minimum"=0.0 ("Data Entry Limits:Minimum")) -> (error out=w286:errorcluster)  [unwired: 1 in, 1 out]
        n95 = To Long Integer(number=w297) -> (32bit integer=w296:i32)
        n96 = call "Get_Preinitialized_Images-1.vi"("error IN"=w295, "[IN] Number of event"=w290, "[IN] Images Array"=w294) -> ("error OUT"=w293:errorcluster, "[OUT] Processed Image #2"=w277:T3, "[OUT] Processed Image #1"=w283:T3, "[OUT] Source Image #1"=w292:T3)  [unwired: 1 in, 1 out]
        n97 = Number To Decimal String(number=w290) -> (decimal integer string=w289:string)  [unwired: 1 in]
        n98 = Bundle(cluster=w300, "Erosion"="# Erosion", "Connectivity"="Connectivity", "Type of particle filter"=w301) -> (w284:T15)
        n99 = property on="Keep Nega-\ntive Values?" class="Bool (strict)"(error in=w286) -> ("Value"=w267:bool)  [unwired: 1 in, 2 out]
        n100 = call "Refresh_Image_by_Copying_Fresh_One-1.vi"("[IN] Image Type"=w271, "[IN] Unique ID\n(# of Event)"=w289, "error IN"=w293, "Frame Number"="# Frame3", "[IN] Preinitialized Image"=w292, "[IN] AVI Refnum"=w291) -> ("error OUT"=w281:errorcluster, "[OUT] Frame"=w285:T3, "[OUT] AVI Refnum"=w272:T9)  [unwired: 1 in]
        n101 = case shown="True" "Find ALL objects" {
          tunnel: w296 -> [_ w329]
          tunnel: w281 -> [w326 w338]
          tunnel: w272 -> [_ w342]
          tunnel: [w326 w332] -> w299
          tunnel: [w327 w330] -> w315
          tunnel: [w325 w331] -> w306
          tunnel: w318 -> [w327 _]
          tunnel: w305 -> [w325 _]
          tunnel: w269 -> [_ w344]
          tunnel: w284 -> [_ w343]
          tunnel: w282 -> [_ w341]
          tunnel: w271 -> [_ w340]
          tunnel: w270 -> [_ w336]
          tunnel: w267 -> [_ w335]
          frame False {
          }
          frame True {
            n102 = call "Initialize_Cluster_Points_Areas-1.vi"("[IN] Number of frames"=w329) -> ("[OUT] Cluster of \npoints and areas"=w339:T18)
            n103 = property on="Progress" class="Slide (strict)"(error in=w338, "Value"=u8 0 ("Progress")) -> ()  [unwired: 1 in, 2 out]
            n104 = Decrement(x=w329) -> (x-1=w328:i32)
            n105 = for {
              N: w329 -> [_]
              tunnel: w344 -> [w349]
              tunnel: w343 -> [w350]
              tunnel: w342 -> [w351]
              tunnel: w341 -> [w355]
              tunnel: w338 -> [w373]
              tunnel: w340 -> [w372]
              tunnel: [w366] -> w333
              shift-right: [w360] -> w334
              shift-left: w339 -> [w362]
              tunnel: w328 -> [w357]
              tunnel: w336 -> [w348]
              tunnel: w335 -> [w345]
              i -> [w359]
              n106 = To Unsigned Long Integer(number=w359) -> (unsigned 32bit integer=w353:u32)
              n107 = Index Array(array=w362, index=w359) -> (element=w365:T19)
              n108 = Number To Decimal String(number=w353) -> (decimal integer string=w374:string)  [unwired: 1 in]
              n109 = call "Initialize_Image_with_Random_Name-3.vi"("error IN"=w373, "Image Type"=w372, "Unique ID"=w374) -> ("error OUT"=w371:errorcluster, "[OUT] New Image"=w352:T3)
              n110 = call "Initialize_Image_with_Random_Name-3.vi"("error IN"=w373, "Image Type"=w372, "Unique ID"=w374) -> ("error OUT"=w370:errorcluster, "[OUT] New Image"=w354:T3)
              n111 = Merge Errors(w371, w370) -> (w356:errorcluster)
              n112 = call "Detect_Particle(Array)-2.vi"("[IN] Sample Image"=w352, "[IN] AVI Refnum"=w351, "[IN] Particle Searching Settings"=w350, "Keep Nega-\ntive Values?"=w345, "[IN] Frame Number"=w353, "[IN] Destination Image"=w354, "[IN] Binarization Settings"=w355, "error IN"=w356, "[IN] # Channel"=w349, "[IN] Filtering Settings"=w348) -> ("[OUT] Particle Reports (Pixels)"=w346:T20, "error OUT"=w347:errorcluster)  [unwired: 4 in]
              n113 = call "Get_Centers_Areas_Info_Particles-1.vi"("[IN] Particle Reports (Pixels)"=w346, "error in"=w347) -> ("[OUT] Array of X,Y"=w364:dbl[], "[OUT] Array of Area"=w363:dbl[], "error out"=w369:errorcluster)  [unwired: 1 out]
              n114 = Bundle(cluster=w365, "Points (X,Y)"=w364, "Areas of points (X,Y)"=w363) -> (w361:T19)
              n115 = call "IMAQ Dispose"("Image"=w352, "error in (no error)"=w369) -> ("error out"=w368:errorcluster)  [unwired: 4 in]
              n116 = call "IMAQ Dispose"("Image"=w354, "error in (no error)"=w369) -> ("error out"=w367:errorcluster)  [unwired: 4 in]
              n117 = call "Progress_Local_For_Loop-1.vi"("[IN] Number of Frames"=w357, "[IN] Current Index"=w359) -> ("[OUT] % progress"=→"Progress":u8)
              n118 = Merge Errors(w368, w367) -> (w366:errorcluster)
              n119 = Replace Array Subset(array=w362, new element=w361, index=w359) -> (w360:T18)
            }
            n120 = call "Save_Points(X-Y)_Areas-2.vi"("error IN"=w333, "[IN] Cluster of \npoints and areas"=w334) -> ("error OUT"=w332:errorcluster, "[OUT] Areas"=w331:dbl[][], "[OUT] Points (X,Y)"=w330:dbl[][])  [unwired: 1 in]
          }
        }
        n121 = call "Detect_Particle-8.vi"("[IN] Filtering Settings"=w270, "Keep Nega-\ntive Values?"=w267, "# Channel"=w269, "Particle Searching Settings"=w284, "error IN"=w281, "Binarization Settings"=w282, "[IN] Destination Image"=w283, "[IN] Frame"=w285) -> ("error OUT"=w280:errorcluster, "[OUT] Particle Reports (Pixels)"=w279:T20, "[OUT] Binarized Image"=→"1st Filtering":T3)  [unwired: 1 in]
        n122 = call "Get_Centers_Areas_Info_Particles-1.vi"("[IN] Particle Reports (Pixels)"=w279, "error in"=w280) -> ("[OUT] Array of X,Y"=w275:dbl[], "error out"=w274:errorcluster)  [unwired: 2 out]
        n123 = call "Paint_Center_of_Particle-7.vi"("[IN] Initialized Image"=w277, "[IN] AVI Refnum"=w272, "[IN] Image Type"=w271, "[IN] Frame Number"="# Frame3", "[IN] Array of X,Y"=w275, "error IN"=w274, "[IN] Filtering Settings"=w270, "Keep Nega-\ntive Values?"=w267, "[IN] # Channel"=w269) -> ("[OUT] Image Dst"=w268:T3, "error OUT"=w273:errorcluster)  [unwired: 5 in]
        "Results on 1st Movie" <- w268
        n124 = Merge Errors(w273, w299) -> (w298:errorcluster)
        n125 = case shown="True" "Save pics (ex)" {
          tunnel: w298 -> [w320 w322]
          tunnel: [w320 w323] -> w309
          tunnel: w268 -> [_ w321]
          frame False {
          }
          frame True {
            n126 = call "SavePics1.vi"("error IN"=w322, "default name"="Proces_Img2", "Image Dst IN"=w321) -> ("error out"=w323:errorcluster)  [unwired: 1 in]
          }
        }
        n127 = Bundle(cluster=w317, "X,Y"=w315, "Areas particles"=w306, "Particle Fil Setups"=w284, "Tracks, Coordinates"=w316) -> (w314:T12)
      }
      event "Tracking Procedure": Value Change {
        n128 = event-data() -> ()  [unwired: 1 in, 1 out]
        n129 = control-ref of="Max angle"() -> (w397:refnum<vi>)
        n130 = control-ref of="Closing gaps"() -> (w399:refnum<vi>)
        n131 = control-ref of="Min TRK L"() -> (w396:refnum<vi>)
        n132 = control-ref of="dR min"() -> (w387:refnum<vi>)
        n133 = control-ref of="dR max"() -> (w386:refnum<vi>)
        n134 = control-ref of="% linearity"() -> (w398:refnum<vi>)
        n135 = call "Buttons_Limits(Tracking_Page)-1.vi"("[IN] dR max"=w386, "[IN] % linearity"=w398, "[IN] dR min"=w387, "[IN] Min TRK L"=w396, "error IN"=w401, "[IN] Number of Frames"=w400, "[IN] Max angle"=w397, "[IN] Closing gaps"=w399) -> ("error OUT"=w382:errorcluster)  [unwired: 3 in]
        n136 = control-ref of="Tracking progress"() -> (w389:refnum<vi>)
        n137 = Bundle("dR min"="dR min", "dR max"="dR max", "Closing gaps"="Closing gaps", "Min TRK L"="Min TRK L", "% linearity"="% linearity", "Max angle"="Max angle", "Tracking progress"=w389) -> (w384:T7)  [unwired: 1 in]
        n138 = call "Tracking_SubVI-4.vi"("[IN] Control Parameters"=w384, "error IN"=w382, "[IN] Before-After Tracks"=w383, "[IN] Movie Values"=w380) -> ("error OUT"=w378:errorcluster, "[OUT] Before-After Tracks"=w381:T14, "[OUT] Obtained Movie Values"=w379:T12, "[OUT] Number of \nRaw Displacements"=→"Raw #":i32)  [unwired: 4 in]
      }
      event "Filter Tracks": Value Change {
        n139 = event-data() -> ()  [unwired: 1 in, 1 out]
        n140 = call "Apply_Filters_to_Tracks-1.vi"("error IN"=w425, "[IN] Control Parameters"=w409, "[IN] Movie Values"=w424) -> ("error OUT"=w417:errorcluster, "[OUT] Filtered Tracks"=w405:T21, "[OUT] # Displ after Filtration"=→"Saved #":i32, "[OUT] Filtered Movie Values"=w415:T12)  [unwired: 5 in]
        n141 = control-ref of="Save pictures"() -> (w419:refnum<vi>)
        n142 = control-ref of="Delete Tracs"() -> (w418:refnum<vi>)
        n143 = control-ref of="Raw #"() -> (w422:refnum<vi>)
        n144 = control-ref of="Saved #"() -> (w421:refnum<vi>)
        n145 = control-ref of="Frame"() -> (w420:refnum<vi>)
        n146 = call "Disactivate_Frames_Until_Get_Tracking_Results-1.vi"("Delete Tracs Ref"=w418, "Save pictures Ref"=w419, "error IN"=w417, "Frame Ref"=w420, "Saved #  Ref"=w421, "Raw # Ref"=w422) -> ()  [unwired: 6 in]
        n147 = call "Calculation_Velocities_Statistics-3.vi"("error IN"=w417, "[IN] Velocities and Times"=w416, "[IN] Filtered Tracks"=w405, "[IN] Movie Values"=w415) -> ("error OUT"=w412:errorcluster, "[OUT] Velocities and Times"=w414:T13)  [unwired: 6 in]
      }
      event "dR min", "dR max", "Min TRK L", "Max angle", "% linearity": Value Change {
        n148 = event-data() -> ()  [unwired: 1 in, 1 out]
        n149 = property on="dR min" class="DigNum (strict)"(error in=w431) -> ("Value"=w442:dbl)  [unwired: 1 in, 2 out]
        n150 = property on="dR max" class="DigNum (strict)"(error in=w431) -> ("Value"=w436:dbl)  [unwired: 1 in, 2 out]
        n151 = property on="Max angle" class="DigNum (strict)"(error in=w431) -> ("Value"=w430:dbl)  [unwired: 1 in, 2 out]
        n152 = property on="% linearity" class="DigNum (strict)"(error in=w431) -> ("Value"=w432:i32)  [unwired: 1 in, 2 out]
        n153 = property on="Min TRK L" class="DigNum (strict)"(error in=w431) -> ("Value"=w433:i32)  [unwired: 1 in, 2 out]
        n154 = Unbundle(w444) -> ("Closing gaps"=w435:i32, "Tracking progress"=w434:refnum<vi>)  [unwired: 5 out]
        n155 = Bundle(cluster=w444, "dR min"=w442, "dR max"=w436, "Closing gaps"=w435, "Min TRK L"=w433, "% linearity"=w432, "Max angle"=w430, "Tracking progress"=w434) -> (w428:T7)
      }
      event "Show Distributions", "Bins": Value Change {
        n156 = event-data() -> ()  [unwired: 1 in, 1 out]
        n157 = Unbundle(w457) -> ("Instant Vel 1st"=w456:dbl[], "Path Vel 1st"=w447:dbl[])  [unwired: 4 out]
        n158 = call "StatisticForVelocities1.vi"("Path Vel (1D)"=w447, "Intervals"="Bins", "Instant Vel (1D)"=w456) -> ("StD Path"=→"StD Path":dbl, "mean Path Vel"=→"mean Path Vel":dbl, "All Path Vel"=→"All Path Vel":T5, "All Instant Vel"=→"All Instant Vel":T5, "mean Instant Vel"=→"mean Instant Vel":dbl, "StD Instant"=→"StD Instant":dbl)
      }
      event "Frame", "Delete Tracs", "Save pictures": Value Change {
        w480 = u8 1 ("# channel")
        n159 = event-data() -> ()  [unwired: 1 in, 1 out]
        n160 = Decrement(x=w502) -> (x-1=w506:u32)
        n161 = property on="Frame" class="DigNum (strict)"(error in=w475, "Maximum"=w506, "Minimum"=0.0 ("Data Entry Limits:Minimum")) -> ()  [unwired: 1 in, 2 out]
        n162 = call "Get_Preinitialized_Images-1.vi"("error IN"=w475, "[IN] Number of event"=i8 6, "[IN] Images Array"=w467) -> ("error OUT"=w500:errorcluster, "[OUT] Processed Image #2"=w483:T3, "[OUT] Processed Image #1"=w487:T3, "[OUT] Source Image #2"=w496:T3, "[OUT] Source Image #1"=w498:T3)  [unwired: 1 in]
        n163 = property on="Keep Nega-\ntive Values?" class="Bool (strict)"(error in=w475) -> ("Value"=w478:bool)  [unwired: 1 in, 2 out]
        n164 = call "IMAQ AVI2 Read Frame"("error in (no error)"=w500, "Frame Number"="Frame", "Image"=w498, "AVI Refnum"=w499) -> ("error out"=w488:errorcluster, "Image Out"=w486:T3, "AVI Refnum (duplicate)"=w497:T9)  [unwired: 5 in]
        n165 = call "Localize_Particles-9-2.vi"("Keep Nega-\ntive Values?"=w478, "# channel"=w480, "error IN"=w488, "[IN] Filtering Settings"=w482, "[IN] Destination Image"=w487, "[IN] Frame"=w486) -> ("error OUT"=w485:errorcluster, "[OUT] LoG Processed Image"=w468:T3)  [unwired: 1 in, 1 out]
        n166 = Unbundle(w508) -> ("Tracks, Coordinates"=w504:T16)  [unwired: 3 out]
        n167 = call "IMAQ AVI2 Read Frame"("error in (no error)"=w485, "Frame Number"="Frame", "Image"=w496, "AVI Refnum"=w497) -> ("error out"=w481:errorcluster, "Image Out"=w484:T3)  [unwired: 5 in, 1 out]
        n168 = Unbundle(w504) -> ("(X,Y,dX,dY) NN filtered"=w469:dbl[][], "(X,Y,dX,dY) TH filtered"=w494:dbl[][])  [unwired: 5 out]
        n169 = call "Localize_Particles-9-2.vi"("Keep Nega-\ntive Values?"=w478, "# channel"=w480, "error IN"=w481, "[IN] Filtering Settings"=w482, "[IN] Destination Image"=w483, "[IN] Frame"=w484) -> ("error OUT"=w473:errorcluster, "[OUT] LoG Processed Image"=w479:T3)  [unwired: 1 in, 1 out]
        n170 = call "Paint_Tracks_on_Frame-1.vi"("Delete \nOverlay?"="Delete Tracs", "[IN] Number of event"=i8 24, "[IN] Images Array"=w467, "error IN"=w473, "# Frame"="Frame", "[IN] #1 Array (X,Y,...)"=w469, "[IN] #1 Processed Image"=w468) -> ("error OUT"=w471:errorcluster, "[OUT] #1 Overlayed Image"=w472:T3)  [unwired: 2 in]
        "1st Filtering (NN)" <- w472
        n171 = call "Paint_Tracks_on_Frame-1.vi"("Delete \nOverlay?"="Delete Tracs", "[IN] Number of event"=i8 21, "[IN] Images Array"=w467, "error IN"=w471, "# Frame"="Frame", "[IN] #1 Array (X,Y,...)"=w494, "[IN] #1 Processed Image"=w479) -> ("error OUT"=w489:errorcluster, "[OUT] #1 Overlayed Image"=w490:T3)  [unwired: 2 in]
        "1st Filtered" <- w490
        n172 = case shown="True" "Save pictures" {
          tunnel: w490 -> [_ w518]
          tunnel: w472 -> [_ w515]
          tunnel: w489 -> [w511 w517]
          tunnel: [w511 w512] -> w509
          frame False {
          }
          frame True {
            n173 = call "SavePics1.vi"("error IN"=w517, "default name"="Track_Img1", "Image Dst IN"=w518) -> ("error out"=w513:errorcluster)  [unwired: 1 in]
            n174 = call "SavePics1.vi"("error IN"=w513, "default name"="Track_Img2", "Image Dst IN"=w515) -> ("error out"=w512:errorcluster)  [unwired: 1 in]
          }
        }
      }
      event "Testing Frame", "Delete Tracs 3", "Save pictures 2", "Tracks group", "Save problem trks": Value Change {
        w527 = u8 1 ("# channel")
        n175 = event-data() -> ()  [unwired: 1 in, 1 out]
        n176 = Unbundle(w523) -> ("Before Grouped Tracks"=w541:T22, "After Grouped Tracks"=w533:T22, "Current\nGroup"=w564:i32)
        n177 = call "Get_Preinitialized_Images-1.vi"("error IN"=w562, "[IN] Number of event"=i8 7, "[IN] Images Array"=w556) -> ("error OUT"=w538:errorcluster, "[OUT] Processed Image #2"=w536:T3, "[OUT] Processed Image #1"=w540:T3, "[OUT] Source Image #2"=w537:T3, "[OUT] Source Image #1"=w542:T3)  [unwired: 1 in]
        n178 = Array Size(array=w541) -> (size(s)=w558:i32)
        n179 = call "Get_Info_Before-After_Tracks-1.vi"("[IN] After Tracks"=w533, "[IN] Tracks group"="Tracks group", "[IN] Before Tracks"=w541) -> ("Maximal Frame\n(finish point all\ntracks)"=w554:i32, "[OUT] Min Start Pos"=w553:i32)
        n180 = Decrement(x=w558) -> (x-1=w557:i32)
        n181 = property on="Tracks group" class="DigNum (strict)"(error in=w538, "Maximum"=w557, "Minimum"=0.0 ("Data Entry Limits:Minimum")) -> (error out=w565:errorcluster)  [unwired: 1 in, 1 out]
        n182 = property on="Keep Nega-\ntive Values?" class="Bool (strict)"(error in=w538) -> ("Value"=w525:bool)  [unwired: 1 in, 2 out]
        n183 = property on="Testing \nFrame" class="DigNum (strict)"(error in=w565, "Maximum"=w554, "Minimum"=w553) -> (error out=w563:errorcluster)  [unwired: 1 in, 1 out]
        n184 = property on="Tracks \ngroup" class="DigNum (strict)"(error in=w563) -> (error out=w559:errorcluster, "Value"=w522:i32)  [unwired: 1 in, 1 out]
        n185 = in-place {
          in-place-border: w522 -> [w570]
          n186 = in-place-cluster #1(w523) -> ()  [unwired: 1 out]
          n187 = in-place-cluster #1("Current\nGroup"=w570) -> (w521:T14)
        }
        n188 = To Unsigned Long Integer(number=w553) -> (unsigned 32bit integer=w552:u32)
        n189 = Equal?(x=w522, y=w564) -> (x = y?=w551:bool)
        n190 = case shown="True" w551 {
          tunnel: w559 -> [w602 w604]
          tunnel: w552 -> [w600 _]
          tunnel: [w601 w604] -> w532
          tunnel: [w600 w603] -> w535
          tunnel: "Testing Frame" -> [_ w603]
          frame False {
            n191 = property on="Testing \nFrame" class="DigNum (strict)"(error in=w602, "Value"=w600) -> (error out=w601:errorcluster)  [unwired: 1 in, 1 out]
          }
          frame True {
          }
        }
        n192 = To Long Integer(number="Testing Frame") -> (32bit integer=w546:i32)
        n193 = case shown="True" w551 {
          tunnel: "Delete Tracs 3" -> [_ w578]
          tunnel: w549 -> [_ w577]
          tunnel: [FALSE ("Delete Tracs 3") w576] -> w530
          tunnel: w548 -> [w571 w575]
          tunnel: [w571 w574] -> w529
          tunnel: w546 -> [_ w573]
          frame False {
          }
          frame True {
            n194 = case shown="False" w578 {
              tunnel: w577 -> [w583 _]
              tunnel: [w580 TRUE ("Delete Tracs 3")] -> w576
              tunnel: w575 -> [w579 _]
              tunnel: [w579 w584] -> w574
              tunnel: w573 -> [_ w584]
              frame False {
                n195 = Select(t=TRUE ("Delete Tracs 3"), s=w583, f=FALSE ("Delete Tracs 3")) -> (s? t:f=w580:bool)
              }
              frame True {
              }
            }
          }
        }
        n196 = call "Paint_Tracks_Before-After-3.vi"("[IN] Frame"=w542, "[IN] Destina\ntion Image"=w540, "[IN] AVI Refnum"=w528, "[IN] # channel"=w527, "[IN] Testing Frame"=w535, "[IN] Tracks group"="Tracks group", "[IN] Grouped Tracks"=w541, "Keep Nega-\ntive Values?"=w525, "error IN"=w532, "[IN] Filtering Settings"=w531, "[IN] Delete Tracs"=w530, "[IN] Additional Index"=w529) -> ("[OUT] Image with\nDisplacements"=w539:T3)  [unwired: 2 in, 1 out]
        "Before" <- w539
        n197 = call "Paint_Tracks_Before-After-3.vi"("[IN] Frame"=w537, "[IN] Destina\ntion Image"=w536, "[IN] AVI Refnum"=w528, "[IN] # channel"=w527, "[IN] Testing Frame"=w535, "[IN] Tracks group"="Tracks group", "[IN] Grouped Tracks"=w533, "Keep Nega-\ntive Values?"=w525, "error IN"=w532, "[IN] Filtering Settings"=w531, "[IN] Delete Tracs"=w530, "[IN] Additional Index"=w529) -> ("[OUT] Image with\nDisplacements"=w526:T3)  [unwired: 2 in, 1 out]
        "After" <- w526
        n198 = case shown="True" "Save problem trks" {
          tunnel: w532 -> [_ w598]
          tunnel: w528 -> [_ w592]
          tunnel: "Tracks group" -> [_ w591]
          tunnel: w541 -> [_ w599]
          tunnel: "Save problem trks" -> [_ w590]
          tunnel: "Tracks_Before_Filt" ("default name") -> [_ w597]
          tunnel: w533 -> [_ w595]
          tunnel: "Tracks_After_Filt" ("default name") -> [_ w587]
          tunnel: w531 -> [_ w594]
          tunnel: w525 -> [_ w596]
          tunnel: w525 -> [_ w586]
          frame False {
          }
          frame True {
            w593 = u8 1 ("# channel")
            w588 = u32 2 ("FPS")
            n199 = call "Save_Before-After_Tracks-3.vi"("[IN] Grouped tracks"=w599, "[IN] Filtering Settings"=w594, "# channel"=w593, "[IN] AVI Refnum"=w592, "[IN] Tracks group"=w591, "Save movies?"=w590, "error IN"=w598, "default name"=w597, "[IN] FPS"=w588, "Keep Nega-\ntive Values?"=w596) -> ("error OUT"=w589:errorcluster)  [unwired: 5 in]
            n200 = call "Save_Before-After_Tracks-3.vi"("[IN] Grouped tracks"=w595, "[IN] Filtering Settings"=w594, "# channel"=w593, "[IN] AVI Refnum"=w592, "[IN] Tracks group"=w591, "Save movies?"=w590, "error IN"=w589, "default name"=w587, "[IN] FPS"=w588, "Keep Nega-\ntive Values?"=w586) -> ()  [unwired: 5 in, 1 out]
          }
        }
        n201 = case shown="True" "Save pictures 2" {
          tunnel: w539 -> [_ w608]
          tunnel: w532 -> [w605 w610]
          tunnel: [w605 w609] -> w560
          tunnel: w526 -> [_ w607]
          frame False {
          }
          frame True {
            n202 = Two Button Dialog(message="1 or 2?", 1:"After" ("F button name (\"Cancel\")"), 2:"Before" ("T button name (\"OK\")")) -> (T button?=w612:bool)
            n203 = case shown="False" w612 {
              tunnel: "Trck_ImgN" ("default name") -> [w617 w622]
              tunnel: w610 -> [w618 w621]
              tunnel: [w615 w620] -> w609
              tunnel: w608 -> [_ w619]
              tunnel: w607 -> [w616 _]
              frame False {
                n204 = call "SavePics1.vi"("error IN"=w618, "default name"=w617, "Image Dst IN"=w616) -> ("error out"=w615:errorcluster)  [unwired: 1 in]
              }
              frame True {
                n205 = call "SavePics1.vi"("error IN"=w621, "default name"=w622, "Image Dst IN"=w619) -> ("error out"=w620:errorcluster)  [unwired: 1 in]
              }
            }
          }
        }
      }
      event "Save movies": Value Change {
        # "FPS"
        n206 = event-data() -> ()  [unwired: 1 in, 1 out]
        n207 = Unbundle(w640) -> ("Tracks, Coordinates"=w639:T16)  [unwired: 3 out]
        n208 = Unbundle(w639) -> ("(X,Y,dX,dY) TH filtered"=w635:dbl[][])  [unwired: 6 out]
        n209 = call "Save_Tracking_Results_Movie-2.vi"("Save movies"="Save movies", "FPS"=u32 3 ("Frames Per Second"), "# codec"=4, "error IN"=w636, "AVI Refnum"=w633, "default name"="Processed_Movie1", "(X,Y,dX,dY)"=w635) -> ("error out"=w626:errorcluster)  [unwired: 4 in]
      }
      event "Save data": Value Change {
        n210 = event-data() -> ()  [unwired: 1 in, 1 out]
        n211 = Unbundle(w655) -> ("Instant Vel 1st"=w649:dbl[], "Path Vel 1st"=w654:dbl[])  [unwired: 4 out]
        n212 = case shown="True" "Save data" {
          tunnel: w654 -> [_ w660]
          tunnel: w653 -> [w658 w672]
          tunnel: [w658 w659] -> w646
          tunnel: w649 -> [_ w669]
          tunnel: w644 -> [_ w665]
          frame False {
          }
          frame True {
            n213 = call "File Dialog"("start path"=w665, "default name"="Instant_Velocities", "error in"=w672, "pattern (all files)"="*.csv") -> ("selected path"=w673:path, "error out"=w666:errorcluster)  [unwired: 8 in, 2 out]
            n214 = call-poly <vilib>:"Write To Spreadsheet File.vi"("delimiter (\\t)"="\\t" ("delimiter (\\t)"), "transpose? (no:F)"=TRUE, "format (%.3f)"="%.1f", "1D data"=w669, "file path (dialog if empty)"=w673) -> ()  [unwired: 3 in, 1 out]
            n215 = call "File Dialog2"("start path"=w665, "default name"="Path_Velocities", "error in"=w666, "pattern (all files)"="*.csv") -> ("selected path"=w661:path, "error out"=w659:errorcluster)  [unwired: 8 in, 2 out]
            n216 = call-poly <vilib>:"Write To Spreadsheet File.vi"("delimiter (\\t)"="\\t" ("delimiter (\\t)"), "transpose? (no:F)"=TRUE, "format (%.3f)"="%.1f", "1D data"=w660, "file path (dialog if empty)"=w661) -> ()  [unwired: 3 in, 1 out]
          }
        }
      }
      event "STOP Program": Value Change {
        n217 = event-data() -> ()  [unwired: 1 in, 1 out]
        n218 = Index Array(array=w687, index=0) -> (element=w681:T3)
        n219 = call "IMAQ AVI2 Close"("error in (no error)"=w683, "AVI Refnum"=w684) -> ("error out"=w680:errorcluster)  [unwired: 9 in]
        n220 = call "IMAQ Dispose"("All Images? (No)"=TRUE, "Image"=w681, "error in (no error)"=w680) -> ("error out"=w679:errorcluster)  [unwired: 3 in]
      }
      event Timeout {
        n221 = event-data() -> ()  [unwired: 1 in, 1 out]
      }
    }
    "error out" <- w83
    n222 = Unbundle(w83) -> ("code"=w90:i32, "source"=w89:string)  [unwired: 1 out]
    n223 = call <vilib>:"Simple Error Handler.vi"("error code (no error:0)"=w90, "error source (\" \")"=w89, "error in (no error)"=w83) -> ()  [unwired: 2 in, 5 out]
  }
